vi "main OP600_V2.vi"() -> ()   [LabVIEW 2020]
uses:
  SubVI/OP600ZP_state.ctl
  <userlib>/PCAN Basic/Controls/BaudrateEenum.ctl
  <userlib>/PCAN Basic/Controls/Channel.ctl
  <userlib>/Alex.vi/FGV.ctl
  <vilib>/QMT/GDataBase for MySQL(tm)/MySQL/public/controls/DateType.ctl
  daa43a20-d466-48a4-bfb3-52e05527ce28.vi
  654b273e-591c-4045-8098-318fb337c7b6.vi
  e0de2198-bc36-4bc8-b1fb-14dde5ea0bb3.vi
  a5648d77-eeaa-4b2b-abe7-0ffab4b6f7d7.vi
  f79284c3-d1eb-48d9-b152-1e69b32bb97c.vi
  9714de12-b8a4-46e9-98c0-2b399b9db653.vi
  22d400d8-53c2-4810-82ae-66a3a2ac2ba8.vi
  51409799-00e2-4034-9917-3b3013219290.vi
  4ce1676d-84e0-48fa-8ffd-701686323251.vi
  OP500/VG/VG_progressBar.vi
  OP500/VG/VG_branche.vi
  SubVI/CheminDeBase.vi
  <vilib>/Utility/error.llb/Error Cluster From Error Code.vi
  VG/PN.vi
  VG/PackType.vi
  VG/IS30%.vi
  SubVI/OP600ZP_VGConf.vi
  VG/Ubatt.vi
  VG/OCV.vi
  VG/VG_ALIM.vi
  <vilib>/QMT/GDataBase for MySQL(tm)/MySQL/MySQLConnector.lvclass
  VG/VG_BT3564.vi
  <userlib>/Alex_Peak_lib/PEAK_lib_ALEX.lvlib
  <userlib>/PCAN Basic/PCANBasic.lvlib
panel:
  out "Revision":u32
  out "DeltaV30s":u32
  in  "cluster de sortie 2":T1
  in  "errin":errorcluster
  out "error out":errorcluster
  in  "errin":errorcluster
  in  "O/P/D":i8(slide)=1 scale=0.0..2.0
  out "OFF":bool
  out "PARK":bool=TRUE
  out "DRIVE":bool
  out "ST5520":refnum<visa-resource-name>
  out "BT3564":refnum<visa-resource-name>
  out "ALIM":refnum<visa-resource-name>
  in  "arrêt":bool
  out "BDD":T2
  out "VISA OUT":T3
  out "progression":dbl(slide) scale=0.0..30.0
  out "PN":string
  out "errout 2":errorcluster={"status"=TRUE, "code"=0, "source"="PCAN_CHANNEL ILLEGAL"} caption="errout"
  out "errout":errorcluster caption="sortie d'erreur"
  out "STOP":bool
  out "TOP":string
  out "DRAW":picture
  # "COMMANDE"
  # "DRIVE"
  # "PARK"
  # "OFF"
  # "SCAN ____________________________"
  # "SEALING ____________________________"
  # "CONTI ____________________________"
  # "CAN BAT / VEH ____________________________"
  # "PARK ____________________________"
  # "ISO ____________________________"
  # "OCV ____________________________"
  # "CAPA ____________________________"
  # "PRECHARGE ____________________________"
  # "DCIR ____________________________"
  # "PARK 2  ____________________________"
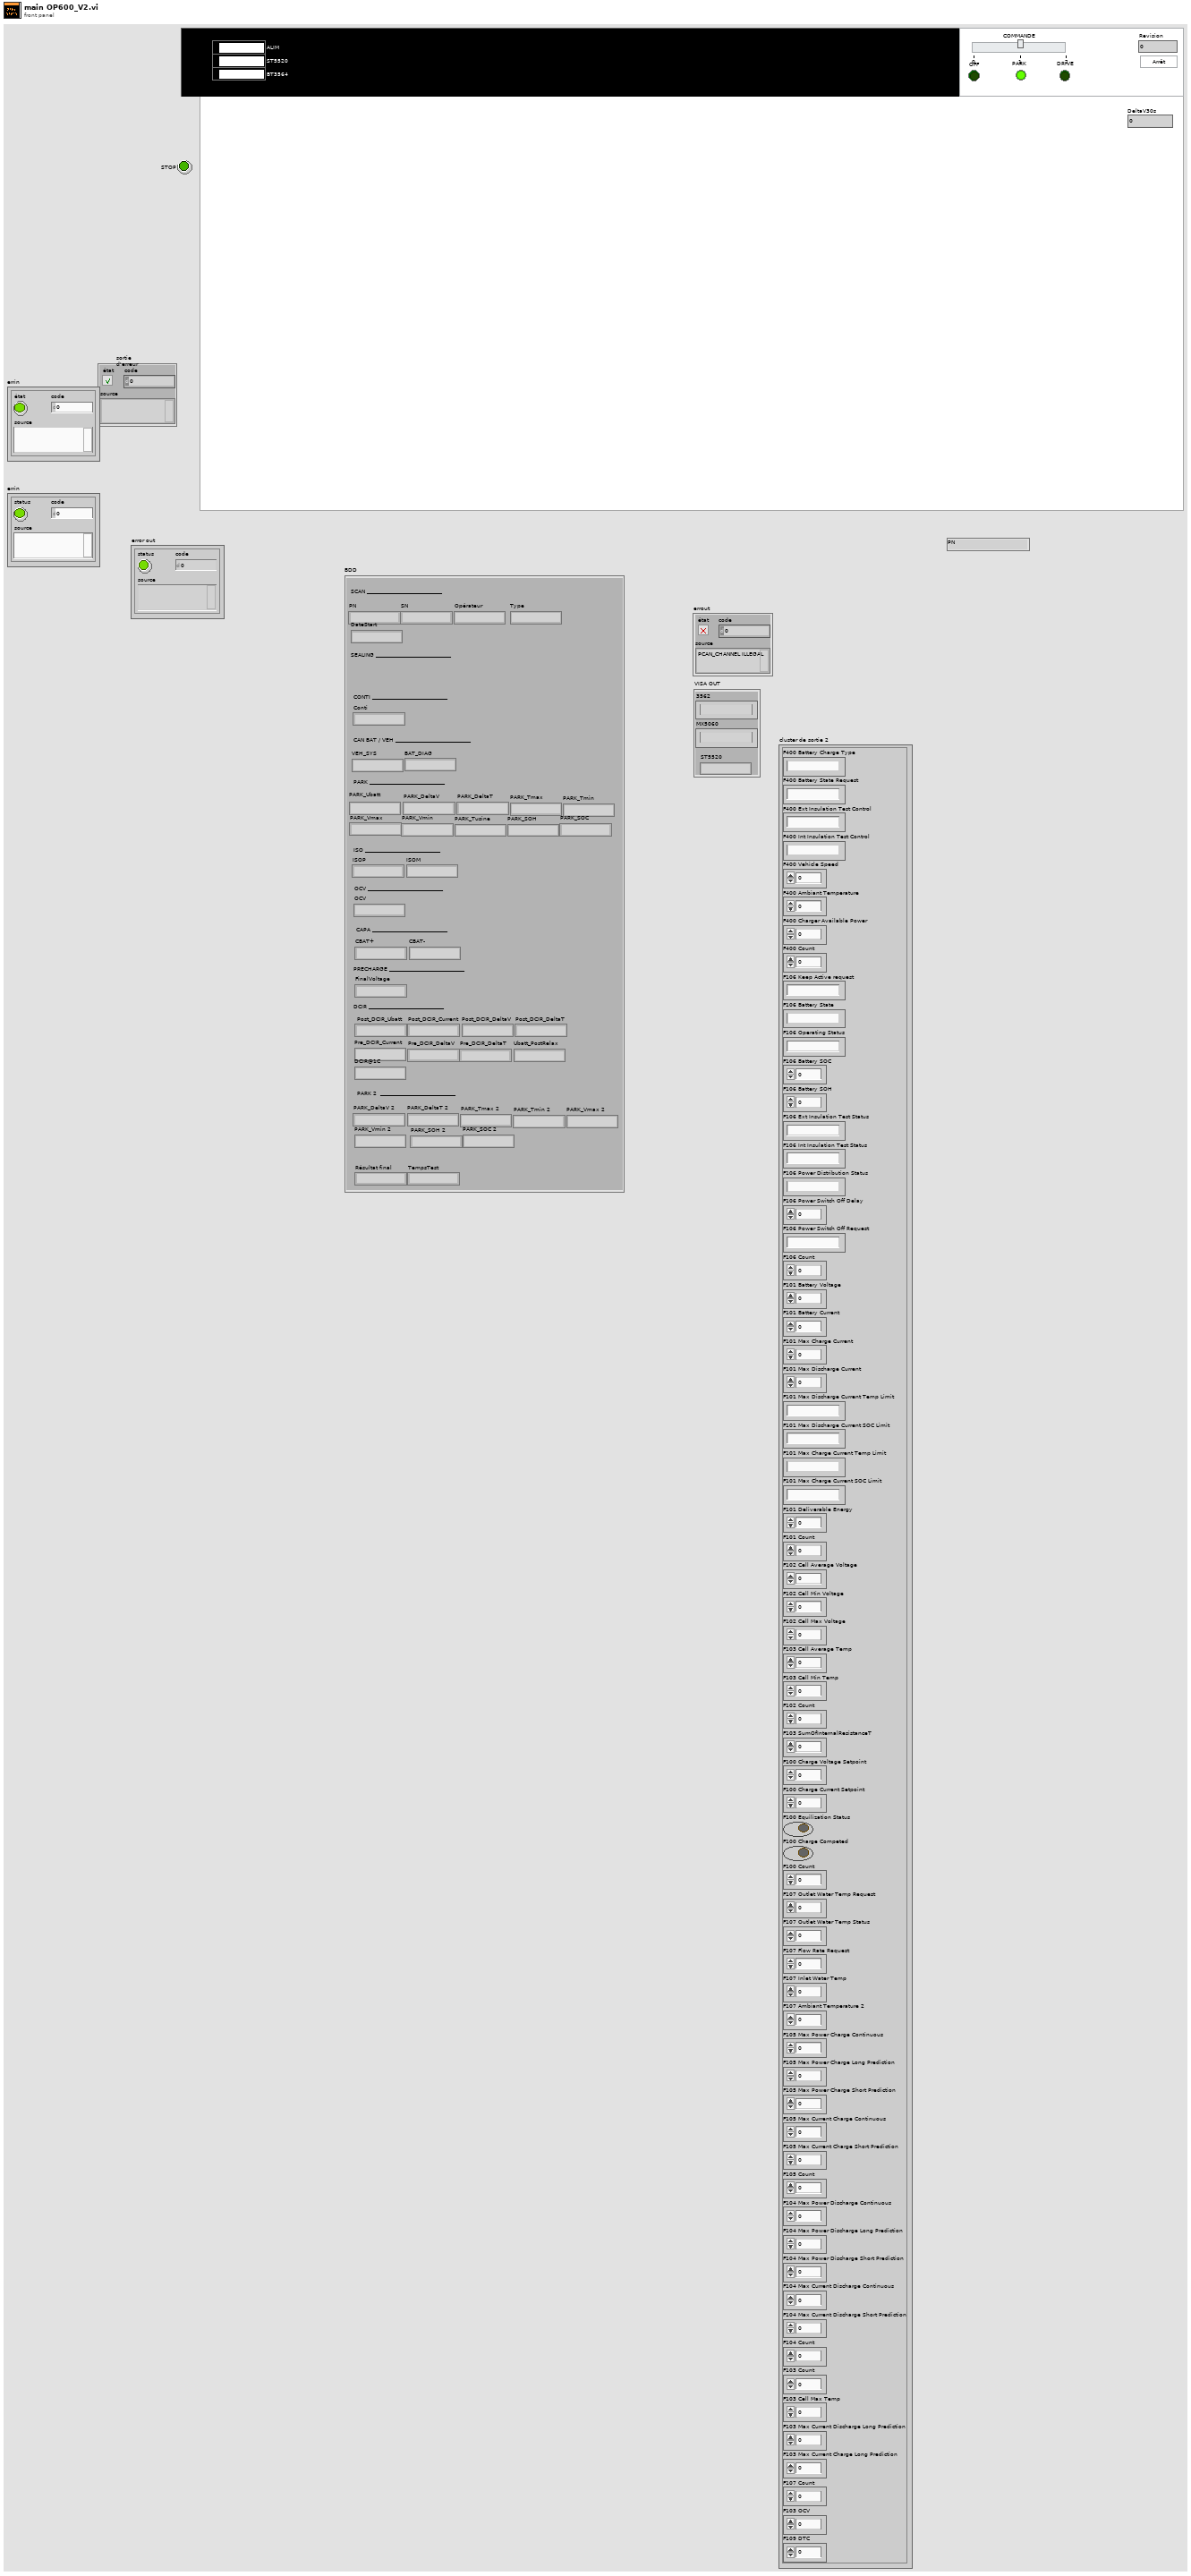
[diagram p1: front panel]
types:
  T1 = cluster{"F400 Battery Charge Type":string, "F400 Battery State Request":string, "F400 Ext Insulation Test Control":string, "F400 Int Insulation Test Control":string, "F400 Vehicle Speed":i32, "F400 Ambiant Temperature":i32, "F400 Charger Available Power":i32, "F400 Count":i32, "F106 Keep Active request":string, "F106 Battery State":string, "F106 Operating Status":string, "F106 Battery SOC":dbl, "F106 Battery SOH":dbl, "F106 Ext Insulation Test Status":string, "F106 Int Insulation Test Status":string, "F106 Power Distribution Status":string, "F106 Power Switch Off Delay":i32, "F106 Power Switch Off Request":string, "F106 Count":i32, "F101 Battery Voltage":u32, "F101 Battery Current":dbl, "F101 Max Charge Current":u32, "F101 Max Discharge Current":u32, "F101 Max Discharge Current Temp Limit":string, "F101 Max Discharge Current SOC Limit":string, "F101 Max Charge Current Temp Limit":string, "F101 Max Charge Current SOC Limit":string, "F101 Deliverable Energy":dbl, "F101 Count":u32, "F102 Cell Average Voltage":u32, "F102 Cell Min Voltage":u32, "F102 Cell Max Voltage":u32, "F103 Cell Average Temp":i32, "F103 Cell Min Temp":i32, "F102 Count":u32, "F103 SumOfInternalResistanceT":i32, "F100 Charge Voltage Setpoint":i32, "F100 Charge Current Setpoint":dbl, "F100 Equilization Status":bool, "F100 Charge Competed":bool, "F100 Count":i32, "F107 Outlet Water Temp Request":i32, "F107 Outlet Water Temp Status":i32, "F107 Flow Rate Request":i32, "F107 Inlet Water Temp":i32, "F107 Ambiant Temperature 2":i32, "F105 Max Power Charge Continuous":i32, "F105 Max Power Charge Long Prediction":i32, "F105 Max Power Charge Short Prediction":i32, "F105 Max Current Charge Continuous":i32, "F105 Max Current Charge Short Prediction":i32, "F105 Count ":i32, "F104 Max Power Discharge Continuous":i32, "F104 Max Power Discharge Long Prediction":i32, "F104 Max Power Discharge Short Prediction":i32, "F104 Max Current Discharge Continuous":i32, "F104 Max Current Discharge Short Prediction":i32, "F104 Count ":i32, "F103 Count":i32, "F103 Cell Max Temp":i32, "F103 Max Current Discharge Long Prediction":i32, "F103 Max Current Charge Long Prediction":i32, "F107 Count":i32, "F103 OCV":i32, "F109 DTC":i32}
  T2 = cluster{"PN":string, "SN":string, "Opérateur":string, "Type":string, "DateStart":string, "Conti":string, "VEH_SYS":string, "BAT_DIAG":string, "PARK_Ubatt":string, "PARK_DeltaV":string, "PARK_DeltaT":string, "PARK_Tmax":string, "PARK_Tmin":string, "PARK_Vmax":string, "PARK_Vmin":string, "PARK_Tusine":string, "PARK_SOH":string, "PARK_SOC":string, "ISOP":string, "ISOM":string, "OCV":string, "CBAT+":string, "CBAT-":string, "FinalVoltage":string, "Post_DCIR_Ubatt":string, "Post_DCIR_Current":string, "Post_DCIR_DeltaV":string, "Post_DCIR_DeltaT ":string, "Pre_DCIR_Current":string, "Pre_DCIR_DeltaV":string, "Pre_DCIR_DeltaT":string, "Ubatt_PostRelax":string, "DCIR@1C":string, "PARK_DeltaV 2":string, "PARK_DeltaT 2":string, "PARK_Tmax 2":string, "PARK_Tmin 2":string, "PARK_Vmax 2":string, "PARK_Vmin 2":string, "PARK_SOH 2":string, "PARK_SOC 2":string, "Résultat final":string, "TempsTest":string}
  T3 = cluster{"3562":string, "MX5060":string, "ST5520":string}
  T4 = typedef "PCANBasic.lvlib/Channel.ctl" = enum16{"PCAN_NONEBUS", "not used1", "not used2", "not used3", "not used4", "not used5", "not used6", "not used7", "not used8", "not used9", "not used10", "not used11", "not used12", "not used13", "not used14", "not used15", "not used16", "not used17", "not used18", "not used19", "not used20", "not used21", "not used22", "not used23", "not used24", "not used25", "not used26", "not used27", "not used28", "not used29", "not used30", "not used31", "not used32", "PCAN_ISABUS1", "PCAN_ISABUS2", "PCAN_ISABUS3", "PCAN_ISABUS4", "PCAN_ISABUS5", "PCAN_ISABUS6", "PCAN_ISABUS7", "PCAN_ISABUS8", "not used41", "not used42", "not used43", "not used44", "not used45", "not used46", "not used47", "not used48", "PCAN_DNGBUS1", "not used50", "not used51", "not used52", "not used53", "not used54", "not used55", "not used56", "not used57", "not used58", "not used59", "not used60", "not used61", "not used62", "not used63", "not used64", "PCAN_PCIBUS1", "PCAN_PCIBUS2", "PCAN_PCIBUS3", "PCAN_PCIBUS4", "PCAN_PCIBUS5", "PCAN_PCIBUS6", "PCAN_PCIBUS7", "PCAN_PCIBUS8", "not used73", "not used74", "not used75", "not used76", "not used77", "not used78", "not used79", "not used80", "PCAN_USBBUS1", "PCAN_USBBUS2", "PCAN_USBBUS3", "PCAN_USBBUS4", "PCAN_USBBUS5", "PCAN_USBBUS6", "PCAN_USBBUS7", "PCAN_USBBUS8", "Not used89", "Not used90", "Not used91", "Not used92", "Not used93", "Not used94", "Not used95", "Not used96", "PCAN_PCCBUS1", "PCAN_PCCBUS2"}
  T5 = typedef "PCANBasic.lvlib/BaudrateEenum.ctl" = enum16{"CAN_Baud_1M", "CAN_Baud_800K", "CAN_BAUD_500K", "CAN_BAUD_250K", "CAN_BAUD_125K", "CAN_BAUD_100K", "CAN_BAUD_95K", "CAN_BAUD_83K", "CAN_BAUD_50K", "CAN_BAUD_47K", "CAN_BAUD_33K", "CAN_BAUD_20K", "CAN_BAUD_10K", "CAN_BAUD_5K", "User Baudrate"}
  T6 = cluster{"PN":string, "Sealing":string, "Opérateur":string, "Conti":string, "OCV":string, "ISOP":string, "ISOM":string, "1_TCellmin":string, "1_TCellmax":string, "1_VCellmin":string, "1_VCellmax":string, "1_Nbmodule":string, "2_TCellmin":string, "2_TCellmax":string, "2_VCellmin":string, "2_VCellmax":string, "2_Nbmodule":string, "Résultat final":string, "Résultat final 2":string, "2_Nbmodule 2":string, "2_VCellmax 2":string, "2_VCellmin 2":string, "2_TCellmax 2":string, "Résultat final 3":string, "2_Nbmodule 3":string, "2_VCellmax 3":string, "2_VCellmin 3":string, "2_TCellmax 3":string, "2_TCellmin 2":string, "1_Nbmodule 2":string, "Résultat final 4":string, "2_Nbmodule 4":string, "2_VCellmax 4":string, "2_VCellmin 4":string, "2_TCellmax 4":string, "Résultat final 5":string, "2_Nbmodule 5":string, "2_VCellmax 5":string, "Résultat final 6":string, "2_Nbmodule 6":string, "2_VCellmax 6":string, "2_VCellmin 5":string, "2_TCellmax 5":string}
  T7 = typedef "OP600ZP_state.ctl" = enum16{"Null", "Demarrage", "Init", "Scan", "Sealing", "VAT", "Conti", "CAN Resistance", "Softs", "MCU", "Iso", "OCV", "DTC", "PreCharge", "DTC2", "PARK", "FIN_TEST", "PackVoltage", "Capacitance", "INTERLOOP", "Current + DCIR", "DataDyn", "Crash", "Next", "Comext"}
  T8 = typedef "FGV.ctl" = enum16{"GET", "SET", "RAZ"}
  T9 = typedef "imagedata.ctl" = cluster{"image type":i32, "image depth":i32, "image":u8[], "mask":u8[], "colors":u32[], "Rectangle":cluster{"left":i16, "top":i16, "right":i16, "bottom":i16}}
  T10 = typedef "MySQLVIEW.lvlib/MySQLConnector.lvclass/DateType.ctl" = enum16{"DATETIME", "DATE", "TIMESTAMP", "TIME", "YEAR (2 digits)", "YEAR (4 digits)"}
  T11 = cluster{string, string, string, string, string, string, string, string}
  T12 = cluster{"3564":string, "ALIM":string, "ST5520":string}
  T13 = cluster{string, string, string, string, string, string, string, string, string, string}
  T14 = cluster{"F101 Battery Voltage":u32, "F101 Battery Current":dbl, u32, i32, "F101 Battery Current":dbl, u32, i32, "F101 Battery Voltage":u32}
  T15 = cluster{string, string, string, string, string, string, string, string, string}
  T16 = cluster{"ID":u32, "MSGTYPE":u8, "LEN":u8, "DATA[0]":u8, "DATA[1]":u8, "DATA[2]":u8, "DATA[3]":u8, "DATA[4]":u8, "DATA[5]":u8, "DATA[6]":u8, "DATA[7]":u8}
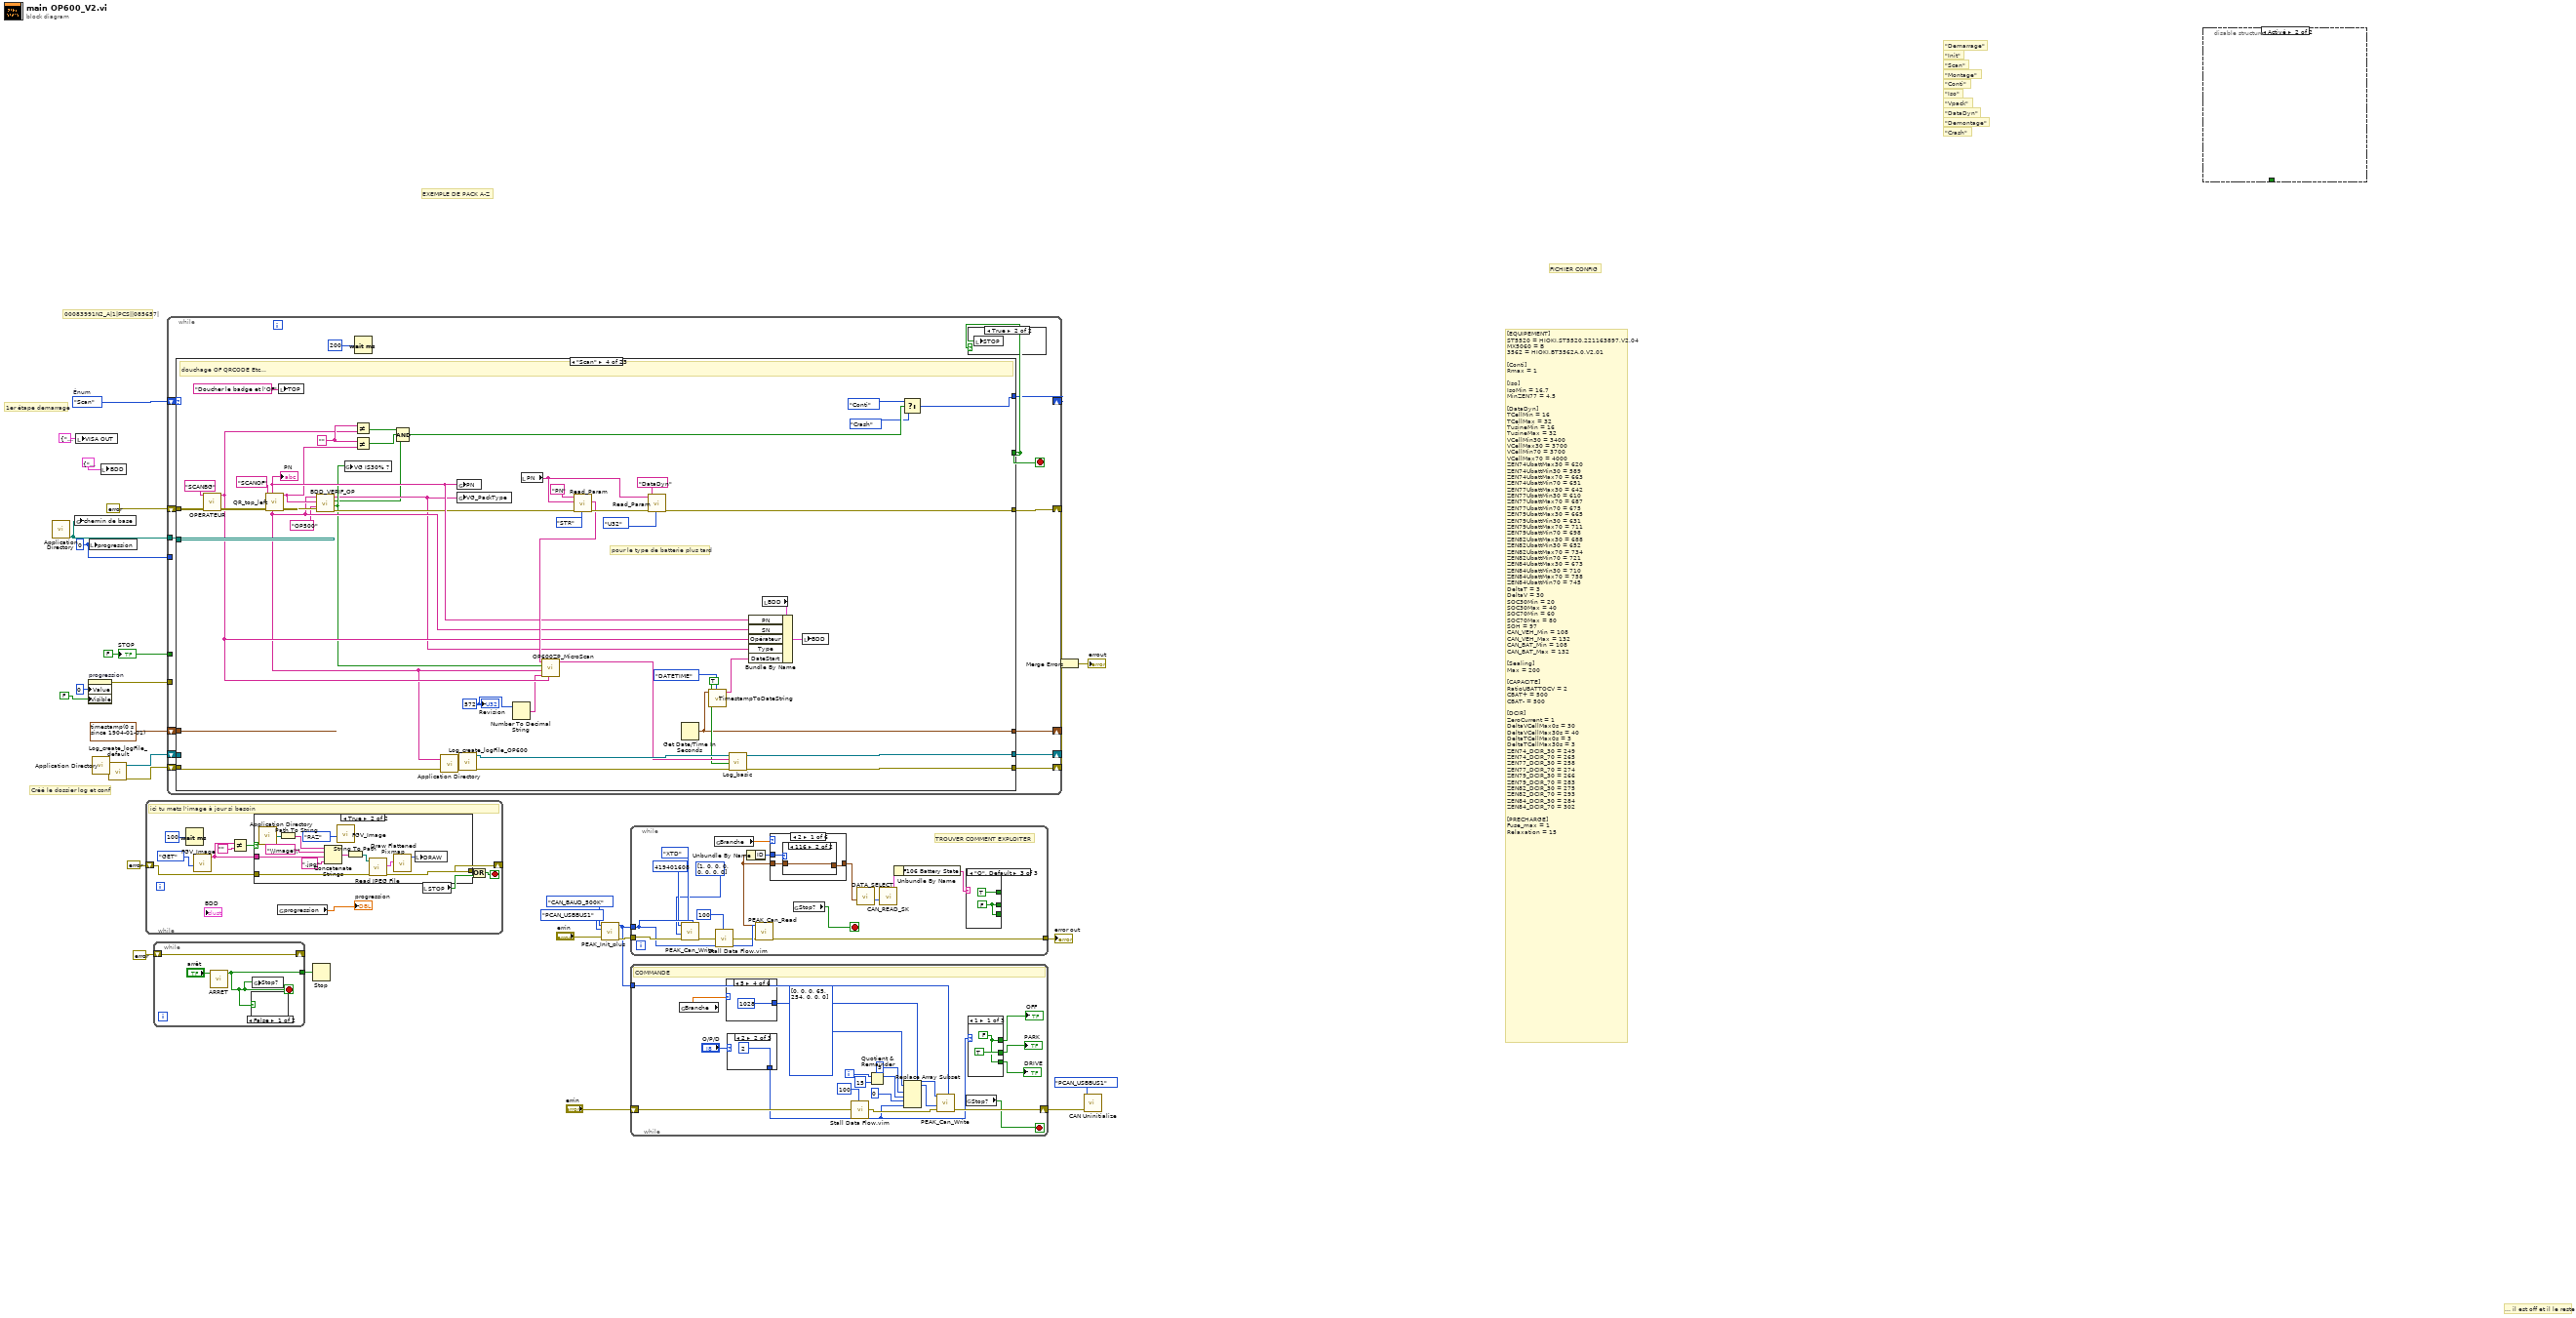
[diagram p0: block diagram]
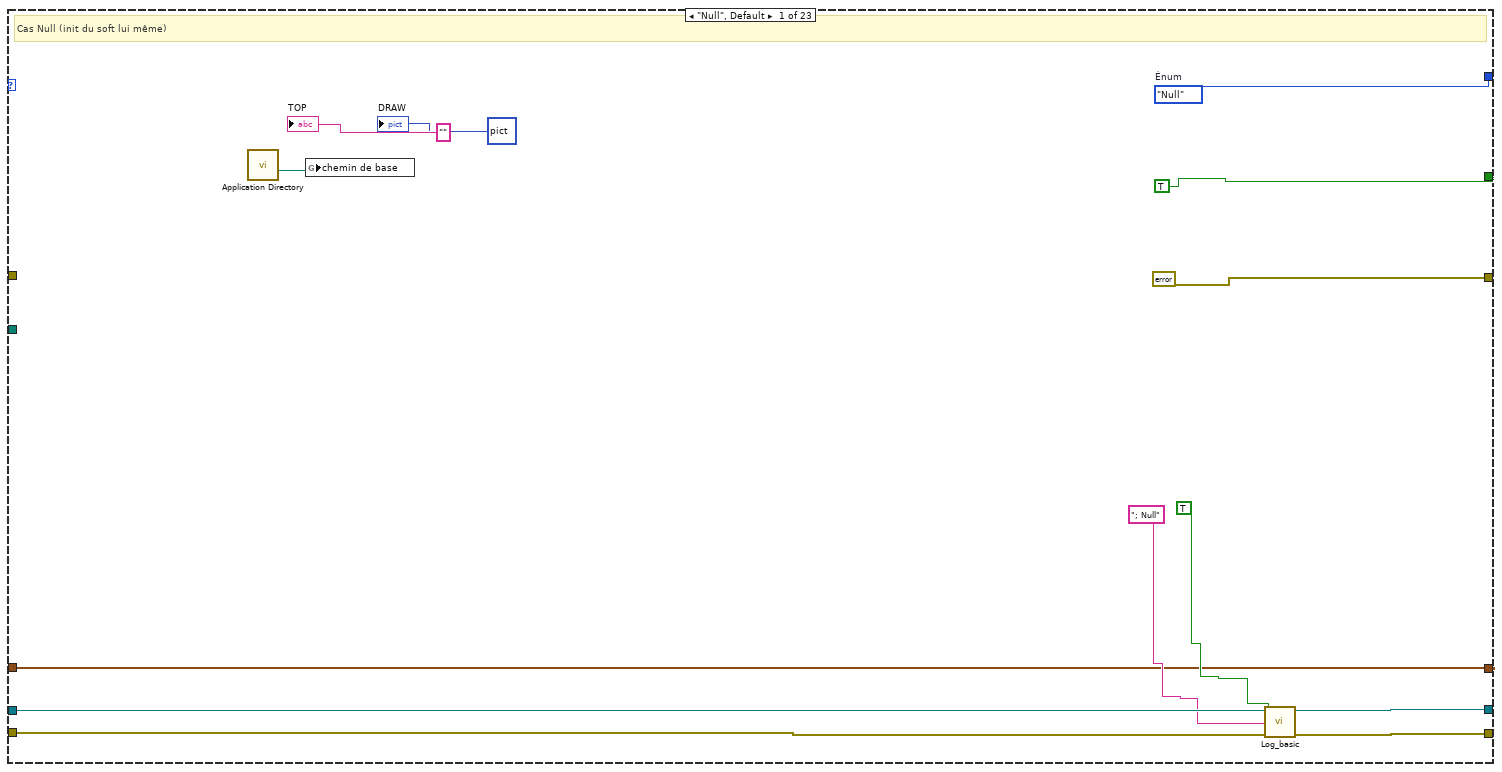
[diagram p2: hidden frame]
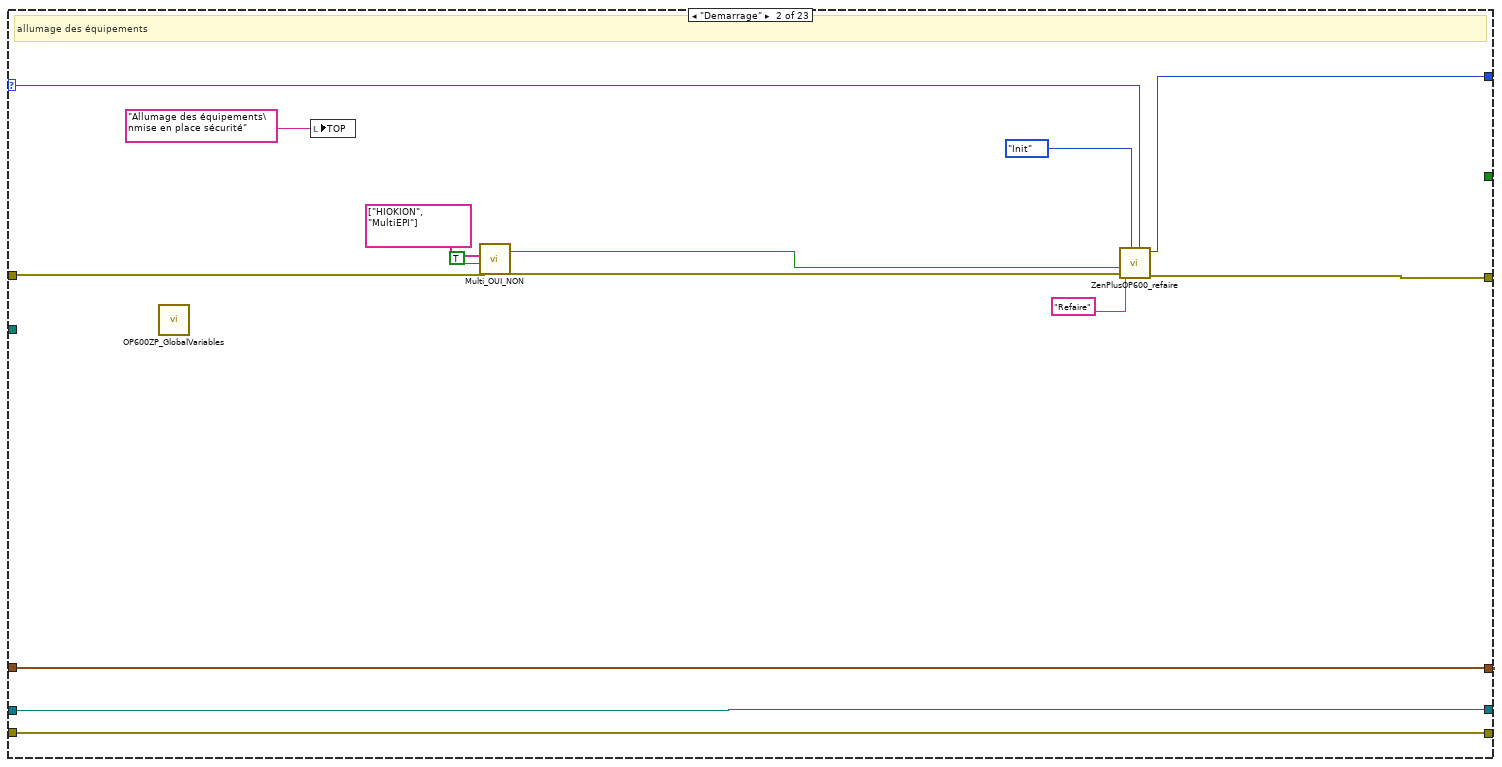
[diagram p3: hidden frame]
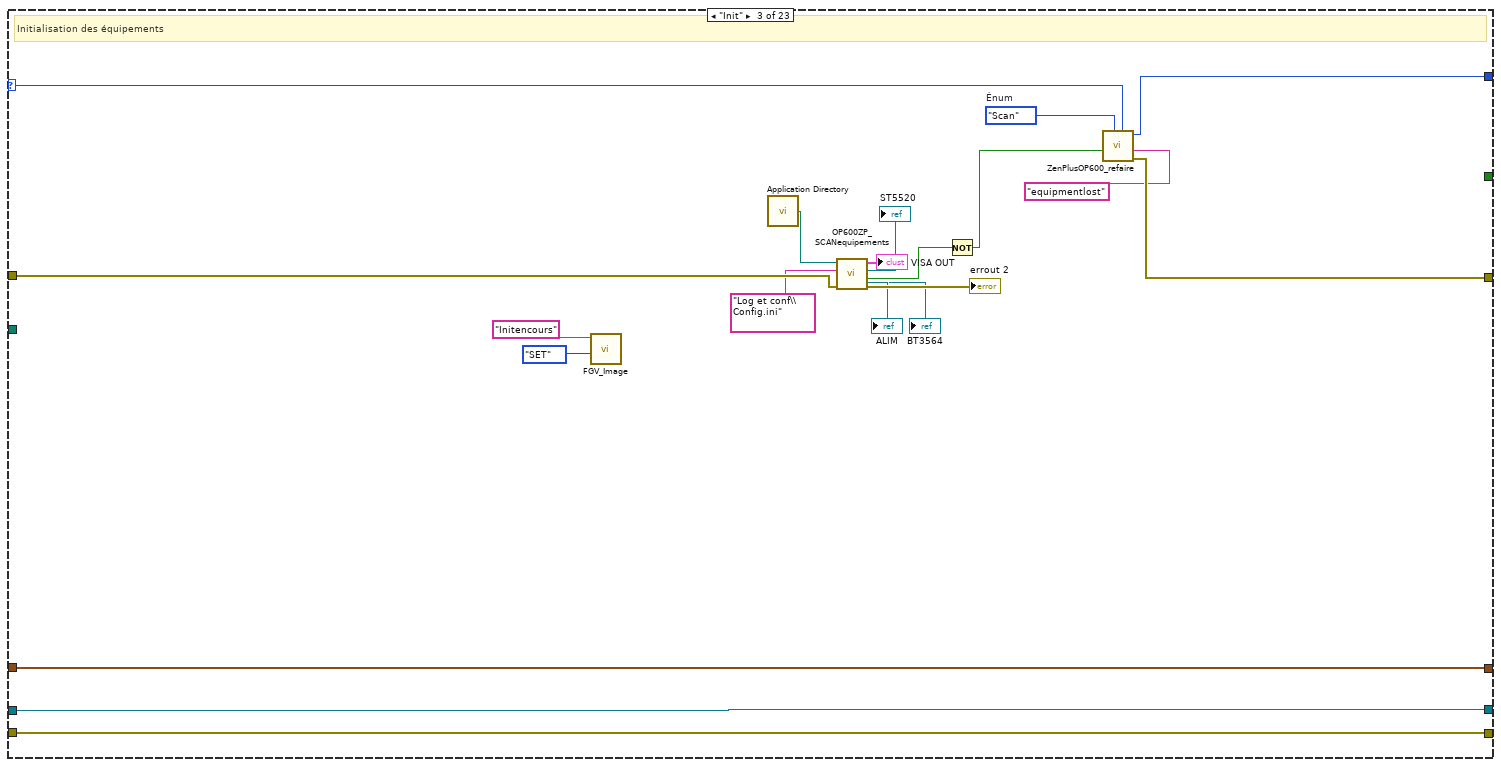
[diagram p4: hidden frame]
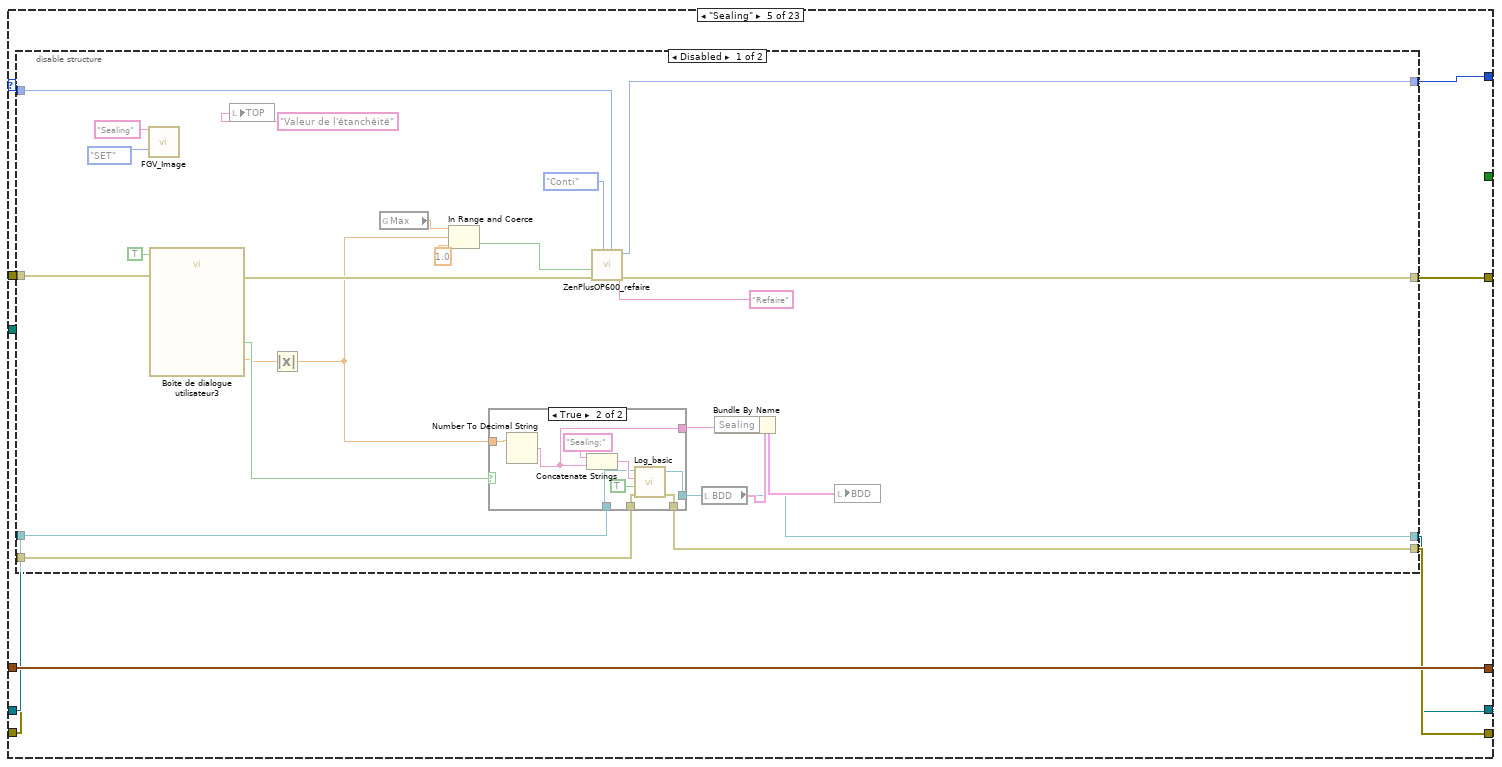
[diagram p5: hidden frame]
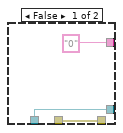
[diagram p6: hidden frame]
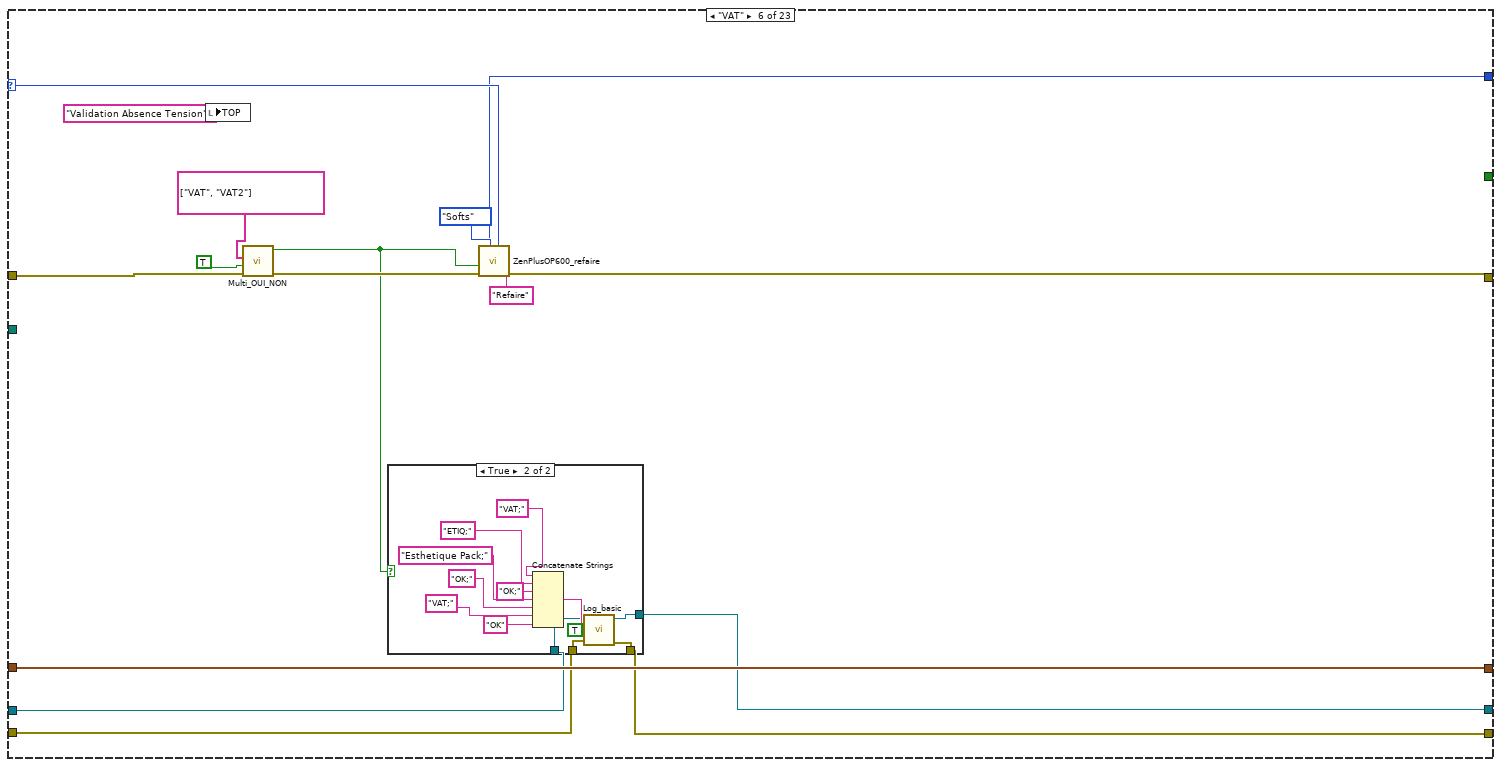
[diagram p8: hidden frame]
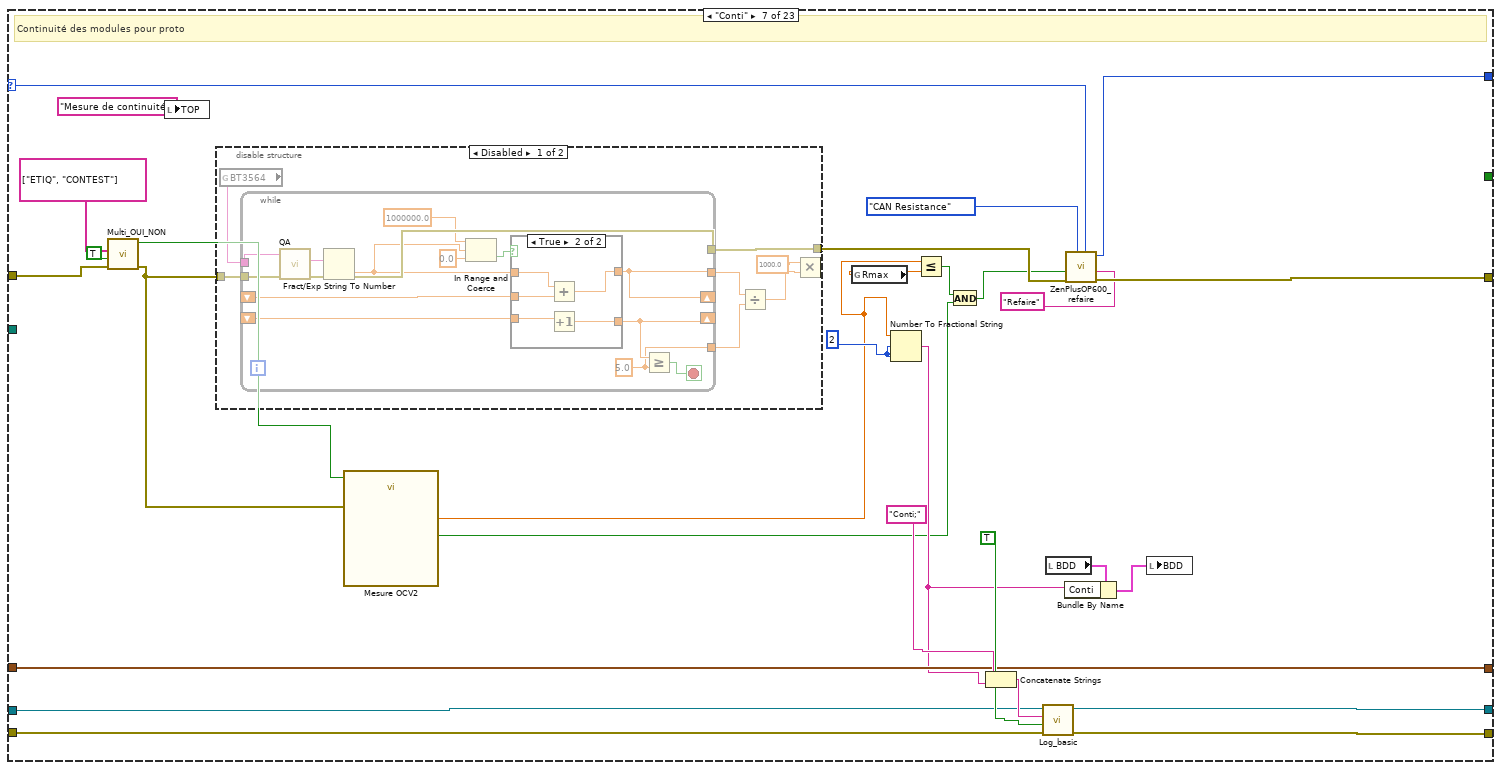
[diagram p10: hidden frame]
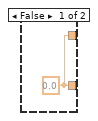
[diagram p11: hidden frame]
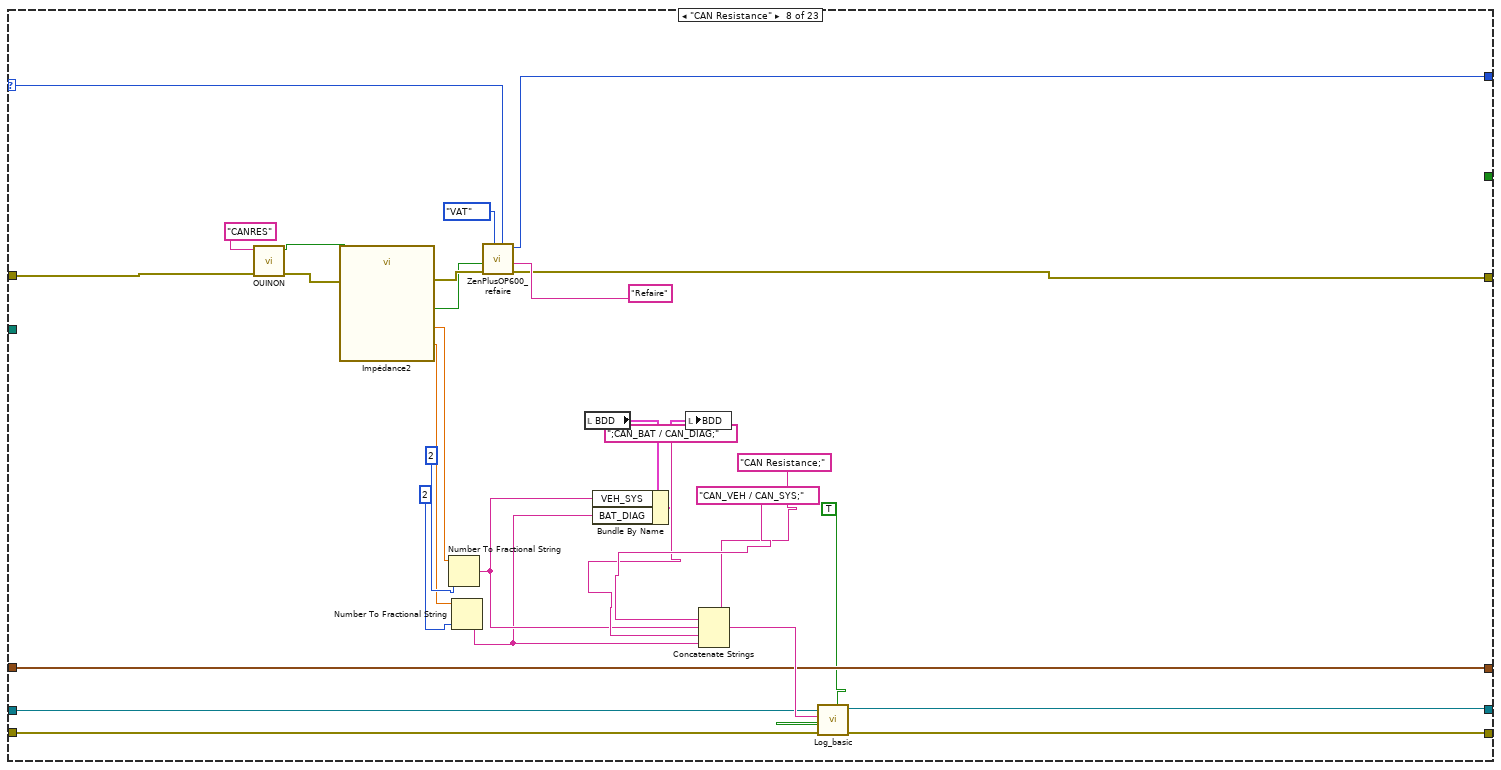
[diagram p13: hidden frame]
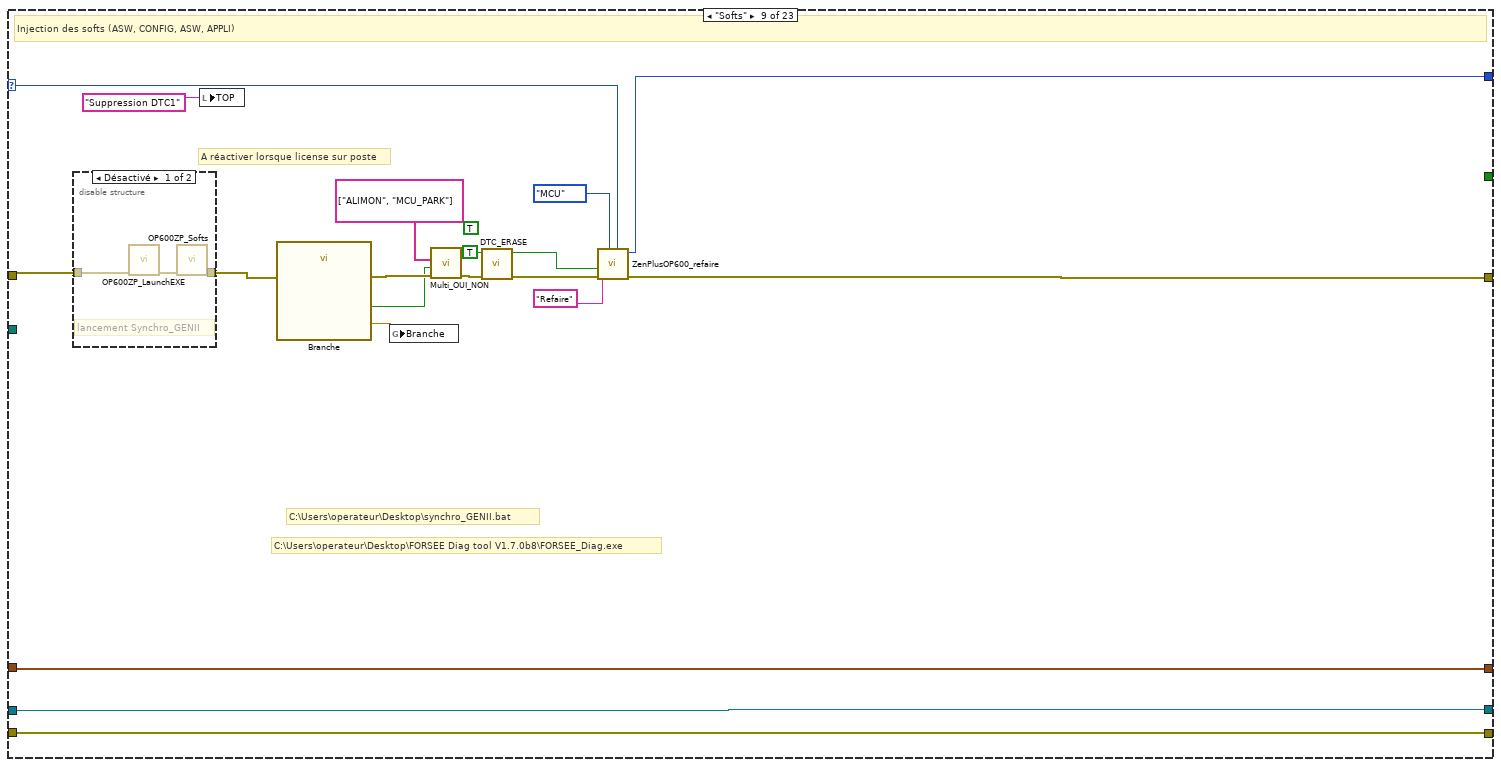
[diagram p14: hidden frame]
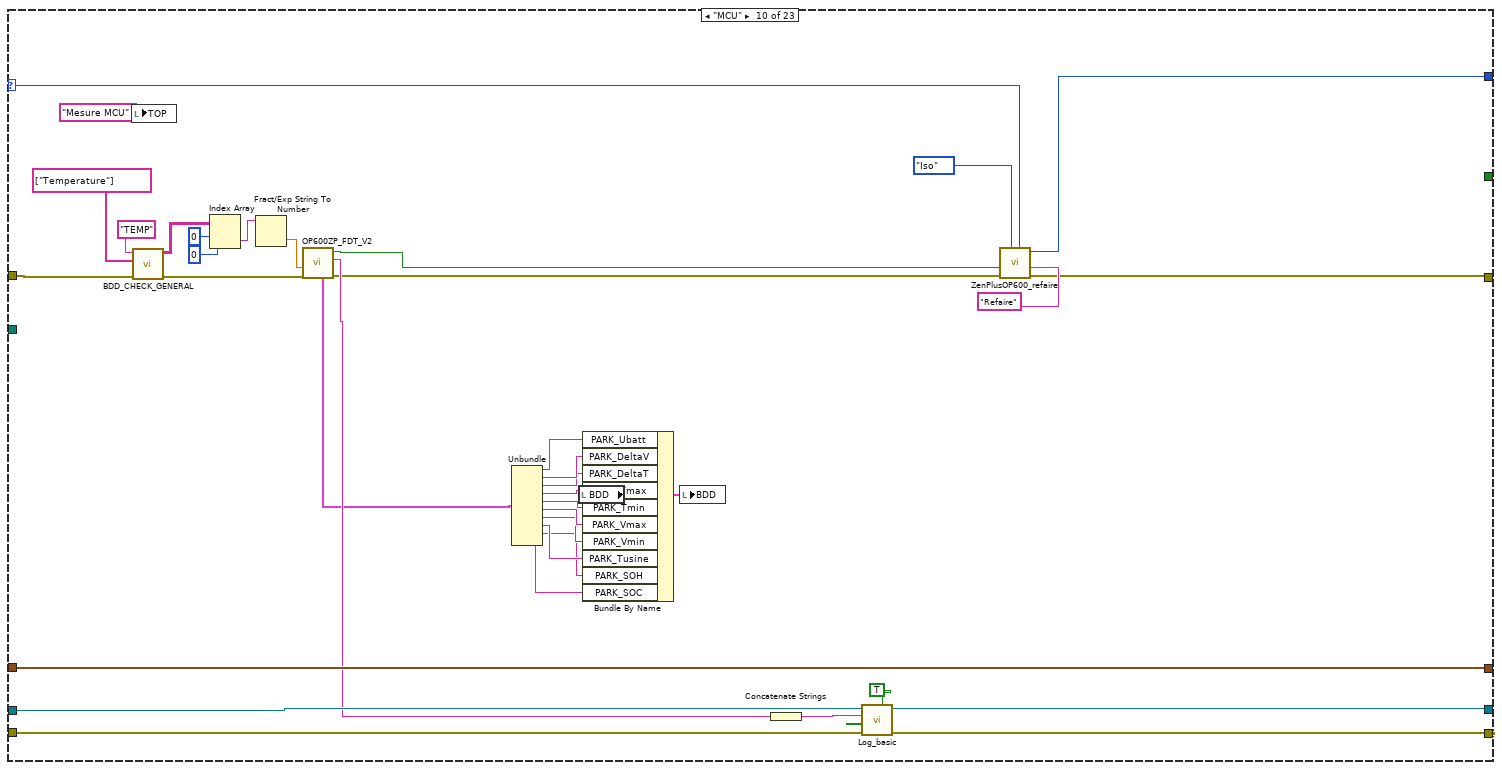
[diagram p16: hidden frame]
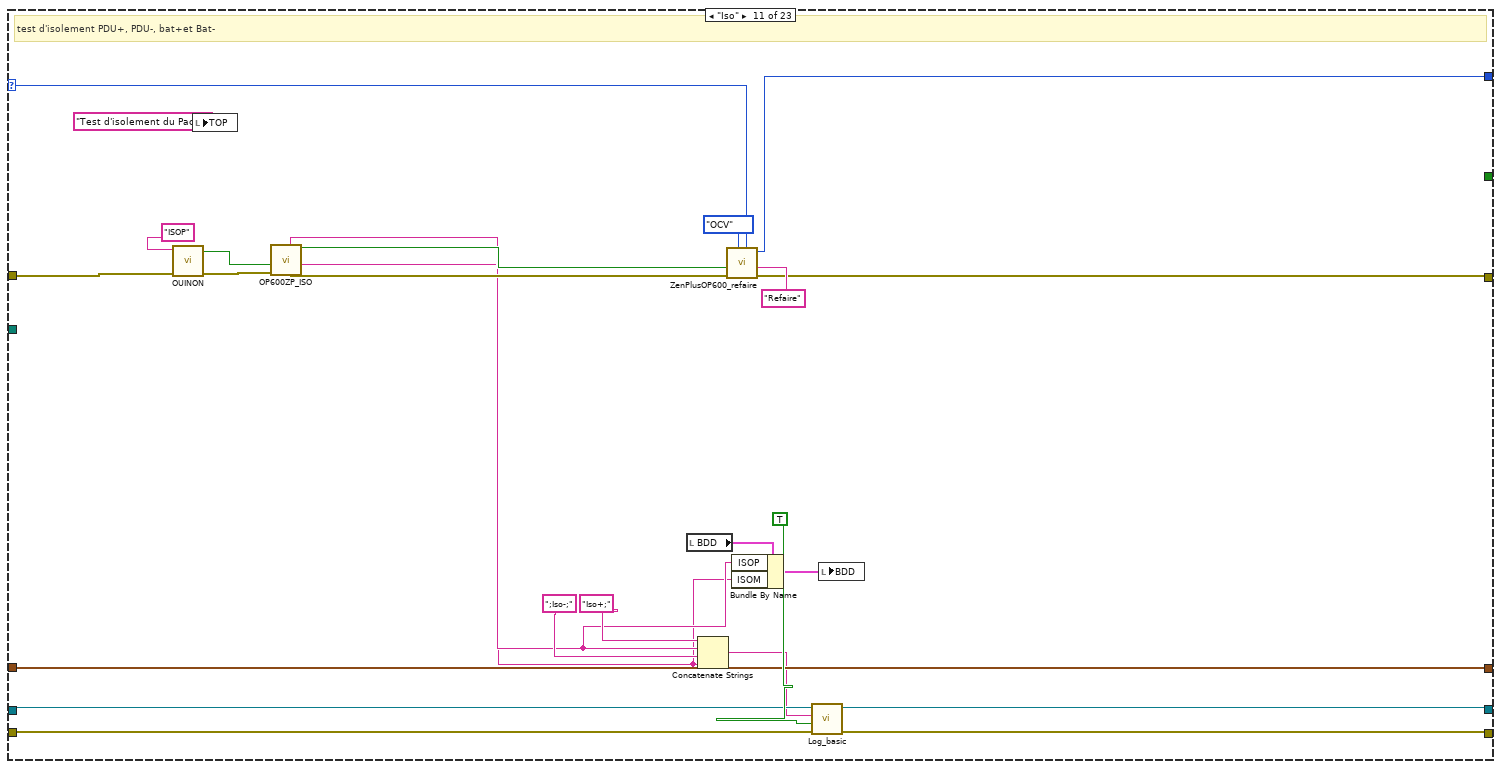
[diagram p17: hidden frame]
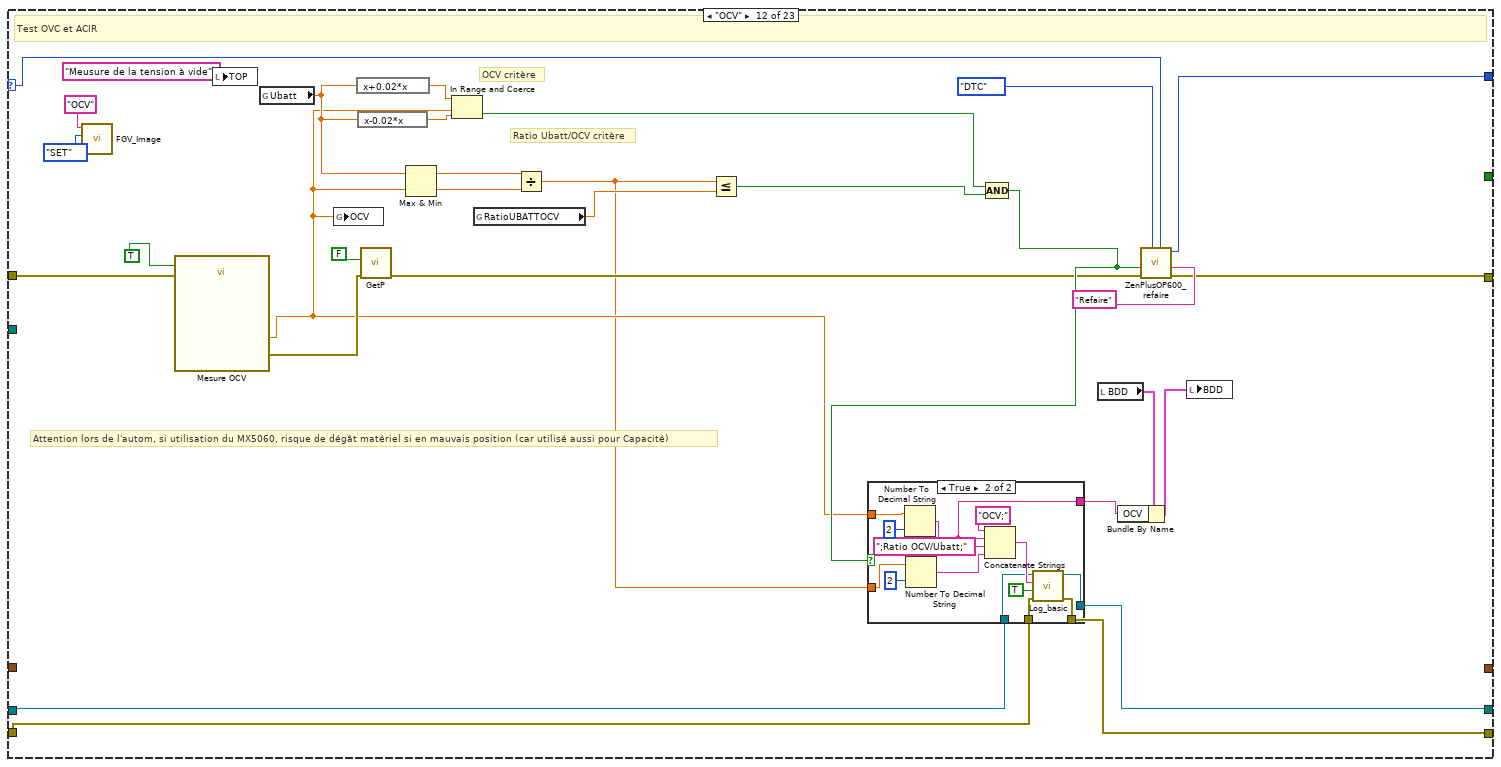
[diagram p18: hidden frame]
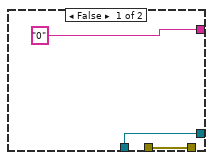
[diagram p19: hidden frame]
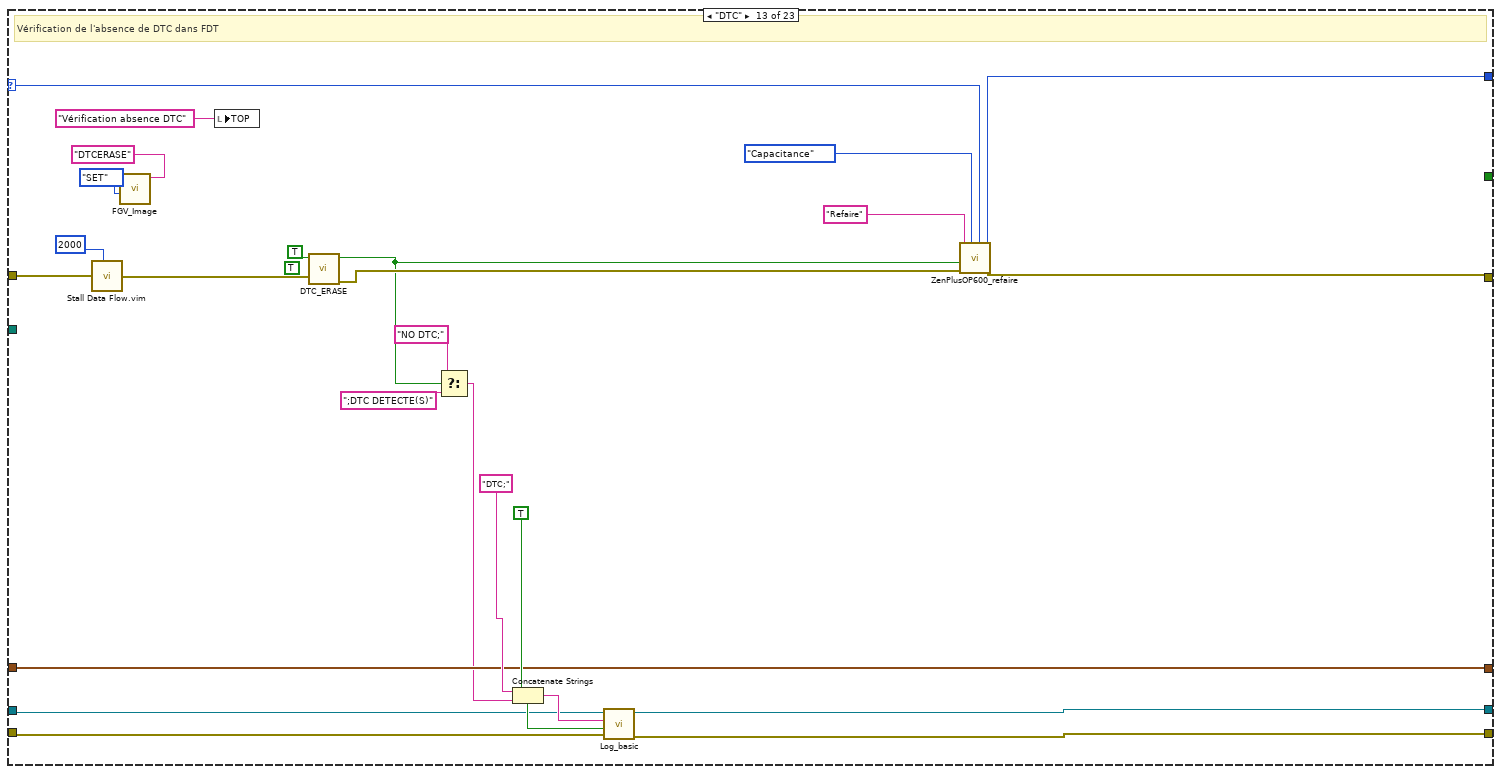
[diagram p20: hidden frame]
diagram:
  w19 = u8 0 ("progression")
  w13 = OP600ZP_state."Scan"  # Énum
  w25 = FALSE ("STOP")
  # "00083991N2_A|1|PCS||085657|"
  # "[EQUIPEMENT]\nST5520 = HIOKI,ST5520,221163897,V2.04\t\nMX5060 = B\n3562 = HIOKI,BT3562A,0,V2.01\n\n[Conti]\nRmax = 1\n\n[Iso]\nIsoMin = 16.7\nMinZEN77 = 4.5\n\n[DataDyn]\nTCellMin = 16\nTCellMax = 32\nTusineMin = 16\nTusineMax = 32\nVCellMin30 = 3400\nVCellMax30 = 3700\nVCellMin70 = 3700\nVCellMax70 = 4000\nZEN74UbattMax30 = 620\nZEN74UbattMin30 = 589\nZEN74UbattMax70 = 663\nZEN74UbattMin70 = 651\nZEN77UbattMax30 = 642\nZEN77UbattMin30 = 610\nZEN77UbattMax70 = 687\nZEN77UbattMin70 = 675\nZEN79UbattMax30 = 665\nZEN79UbattMin30 = 631\nZEN79UbattMax70 = 711\nZEN79UbattMin70 = 698\nZEN82UbattMax30 = 688\nZEN82UbattMin30 = 652\nZEN82UbattMax70 = 734\nZEN82UbattMin70 = 721\nZEN84UbattMax30 = 673\nZEN84UbattMin30 = 710\nZEN84UbattMax70 = 758\nZEN84UbattMin70 = 745\nDeltaT = 3\nDeltaV = 30\nSOC30Min = 20\nSOC30Max = 40\nSOC70Min = 60\nSOC70Max = 80\nSOH = 97\nCAN_VEH_Min = 108\nCAN_VEH_Max = 132\nCAN_BAT_Min = 108\nCAN_BAT_Max = 132\n\n[Sealing]\nMax = 200\n\n[CAPACITE]\nRatioUBATTOCV = 2\nCBAT+ = 500\nCBAT- = 500\n\n[DCIR]\nZeroCurrent = 1\nDeltaVCellMax0s = 30\nDeltaVCellMax30s = 40\nDeltaTCellMax0s = 3\nDeltaTCellMax30s = 3\nZEN74_DCIR_30 = 249\nZEN74_DCIR_70 = 265\nZEN77_DCIR_30 = 258\nZEN77_DCIR_70 = 274\nZEN79_DCIR_30 = 266\nZEN79_DCIR_70 = 283\nZEN82_DCIR_30 = 275\nZEN82_DCIR_70 = 293\nZEN84_DCIR_30 = 284\nZEN84_DCIR_70 = 302\n\n[PRECHARGE]\nFuse_max = 1\nRelaxation = 15"
  # "EXEMPLE DE PACK A-Z"
  # "FICHIER CONFIG"
  # "Créé le dossier log et conf"
  # "1er étape demarrage"
  # "\"Crash\""
  # "\"Demontage\""
  # "\"DataDyn\""
  # "\"Iso\""
  # "\"Montage\""
  # "\"Scan\""
  # "\"Init\""
  # "\"Demarrage\""
  # "\"Conti\""
  # "\"Vpack\""
  # "... il est off et il le reste"
  n1 = call <vilib>:"Application Directory.vi"() -> ("Application Directory"=w24:path)
  n2 = global write "CheminDeBase.vi" "chemin de base"(w24) -> ()
  n3 = local write "VISA OUT"(T3 {"3562"="", "MX5060"="", "ST5520"=""} ("VISA OUT")) -> ()
  n4 = property on="progression" class="Slide (strict)"("Value"=u8 0 ("progression"), "Visible"=FALSE) -> (error out=w17:errorcluster)  [unwired: 2 in, 1 out]
  n5 = local write "progression"(w19) -> ()
  n6 = call <vilib>:"Application Directory.vi"() -> ("Application Directory"=w22:path)
  n7 = local write "BDD"(T6 {"PN"="0", "Sealing"="0", "Opérateur"="0", "Conti"="0", "OCV"="0", "ISOP"="0", "ISOM"="0", "1_TCellmin"="0", "1_TCellmax"="0", "1_VCellmin"="0", "1_VCellmax"="0", "1_Nbmodule"="0", "2_TCellmin"="0", "2_TCellmax"="0", "2_VCellmin"="0", "2_VCellmax"="0", "2_Nbmodule"="0", "Résultat final"="0", "Résultat final 2"="0", "2_Nbmodule 2"="0", "2_VCellmax 2"="0", "2_VCellmin 2"="0", "2_TCellmax 2"="0", "Résultat final 3"="0", "2_Nbmodule 3"="0", "2_VCellmax 3"="0", "2_VCellmin 3"="0", "2_TCellmax 3"="0", "2_TCellmin 2"="0", "1_Nbmodule 2"="0", "Résultat final 4"="0", "2_Nbmodule 4"="0", "2_VCellmax 4"="0", "2_VCellmin 4"="0", "2_TCellmax 4"="0", "Résultat final 5"="0", "2_Nbmodule 5"="0", "2_VCellmax 5"="0", "Résultat final 6"="0", "2_Nbmodule 6"="0", "2_VCellmax 6"="0", "2_VCellmin 5"="0", "2_TCellmax 5"="0"} ("Cluster")) -> ()
  n8 = call <userlib>:"Log_create_logFile_default.vi"("appdir"=w22) -> ("errout"=w23:errorcluster, "Fichier à flux d'octets en sortie"=w26:refnum<file>)  [unwired: 9 in]
  n9 = while {
    shift-right: [w38] -> _
    shift-left: errorcluster {"status"=FALSE, "code"=0, "source"=""} ("error out") -> [w35]
    stop <- w36 stop-if-true
    # "ici tu mets l'image à jour si besoin"
    n10 = Wait (ms)(milliseconds to wait=u32 100 ("attente (ms)")) -> ()  [unwired: 1 out]
    n11 = call <userlib>:"FGV_Image.vi"("Énum"=FGV."GET") -> ("OUT"=w31:string)  [unwired: 10 in]
    n12 = Not Equal?(x=w31, y="") -> (x != y?=w32:bool)
    n13 = case shown="True" w32 {
      tunnel: [w40 w45] -> w38
      tunnel: w35 -> [w40 w44]
      tunnel: w31 -> [_ w43]
      frame False {
      }
      frame True {
        n14 = call <vilib>:"Application Directory.vi"() -> ("Application Directory"=w48:path)
        n15 = Path To String(path=w48) -> (string=w49:string)
        n16 = Concatenate Strings(w49, "\\Image\\" ("chaîne"), w43, ".jpg" ("chaîne")) -> (w47:string)
        n17 = call <userlib>:"FGV_Image.vi"("Énum"=FGV."RAZ") -> ()  [unwired: 10 in, 1 out]
        n18 = String To Path(string=w47) -> (path=w46:path)
        n19 = call <vilib>:"Read JPEG File.vi"("error in (no error)"=w44, "path to JPEG file"=w46) -> ("error out"=w45:errorcluster, "image data"=w52:T9)  [unwired: 7 in, 1 out]
        n20 = call <vilib>:"Draw Flattened Pixmap.vi"("image data"=w52) -> ("new picture"=w41:picture)  [unwired: 8 in]
        n21 = local write "DRAW"(w41) -> ()
      }
    }
    n22 = global read "VG_progressBar.vi" "progression"() -> (→"progression":dbl)
    n23 = local read "STOP"() -> (w37:bool)
    n24 = Or(x=w38, y=w37) -> (x .or. y?=w36:bool)
  }
  n25 = while {
    tunnel: [w53] -> w12
    shift-right: [w54] -> _
    shift-left: errorcluster {"status"=FALSE, "code"=0, "source"=""} ("error out") -> [w54]
    stop <- w53 stop-if-true
    n26 = call "ARRET.vi"("arrêt"="arrêt") -> ("T button?"=w53:bool)  [unwired: 10 in]
    n27 = case shown="False" w53 {
      frame False {
      }
      frame True {
        n28 = call <userlib>:"CAN Uninitialize.vi"() -> ()  [unwired: 9 in, 3 out]
      }
    }
    n29 = global write "VG_Stop" "Stop?"(w53) -> ()
  }
  n30 = while {
    shift-right: [w67] -> w28
    shift-left: errorcluster {"status"=FALSE, "code"=0, "source"=""} ("error out") -> [w58]
    shift-right: [w63] -> w27
    shift-left: w23 -> [w66]
    shift-right: [w64] -> _
    shift-left: w26 -> [w65]
    tunnel: w24 -> [w61]
    tunnel: w25 -> [_]
    shift-right: [w59] -> _
    shift-left: timestamp(0 s since 1904-01-01) ("seconds since 1Jan1904") -> [w60]
    tunnel: w19 -> [_]
    tunnel: w17 -> [_]
    shift-right: [w56] -> _
    shift-left: w13 -> [w57]
    stop <- w62 stop-if-true
    n31 = case shown="\"Scan\"" w57 {
      selector: w57 -> [_ w88 w109 _ w163 w213 w251 w301 w334 w371 w389 w412 w470 w505 w557 w643 w736 w793 w832 w855 _ _ w962]
      tunnel: w58 -> [_ w85 w112 w131 w169 w219 w242 w320 w331 w353 w390 w430 w462 w526 w551 w648 w756 w780 w824 w853 w881 w923 w959]
      tunnel: [errorcluster {"status"=FALSE, "code"=0, "source"=""} ("errin") w90 w111 w147 w161 w211 w256 w298 w335 w374 w394 w429 w479 w506 w555 w644 w737 w785 w816 w849 w880 w927 w961] -> w67
      tunnel: w66 -> [w77 w92 w115 w157 w166 w209 w263 w307 w338 w381 w405 w426 w475 w518 w562 w638 w740 w791 w830 w852 w908 w945 w965]
      tunnel: w65 -> [w78 w95 w114 _ w167 w207 w262 w305 w337 w380 w404 w428 w473 w516 w563 w636 w743 w792 w829 w850 w909 w946 w964]
      tunnel: [w75 w95 w114 w159 w164 w206 w261 w304 w337 w378 w403 w427 w472 w515 w560 w635 w742 w789 w826 w848 _ _ w956] -> w64
      tunnel: [w76 w92 w115 w160 w165 w208 w260 w306 w338 w379 w406 w425 w474 w517 w561 w637 w741 w788 w827 w851 w884 w926 w963] -> w63
      tunnel: [TRUE _ _ _ _ _ _ _ _ _ _ _ _ _ _ _ _ _ _ _ w910 _ _] -> w62
      tunnel: w61 -> [_ _ _ _ _ _ _ _ _ _ _ _ _ _ _ _ _ _ _ _ _ _ w960]
      tunnel: w60 -> [w72 w94 w113 _ w168 w215 w258 w303 w340 w377 w402 _ w471 w513 w559 w641 w757 w790 w828 _ _ _ w957]
      tunnel: [w72 w94 w113 w129 w168 w215 w258 w303 w340 w377 w402 _ w471 w513 w559 w641 w757 w790 w828 _ _ _ w958] -> w59
      tunnel: [w69 w87 w107 w132 w162 w212 w250 w299 w332 w369 w387 w410 w468 w503 w556 w640 w735 w787 w831 w854 OP600ZP_state."Crash" w925 w955] -> w56
      frame "Null", Default {
        w69 = OP600ZP_state."Null"  # Énum
        # "Cas Null (init du soft lui même)"
        n32 = call <vilib>:"Application Directory.vi"() -> ("Application Directory"=w81:path)
        n33 = global write "CheminDeBase.vi" "chemin de base"(w81) -> ()
        n34 = call <userlib>:"Log_basic.vi"("errin"=w77, "date?"=TRUE, "chaîne"="; Null", "in"=w78) -> ("sortie d'erreur"=w76:errorcluster, "refnum en sortie"=w75:refnum<file>)  [unwired: 6 in]
        "DRAW" <- picture data[5B] ("DRAW")
        "TOP" <- "" ("TOP")
      }
      frame "Demarrage" {
        # "allumage des équipements"
        n35 = call "OP600ZP_GlobalVariables.vi"() -> ()  [unwired: 12 in]
        n36 = local write "TOP"("Allumage des équipements\nmise en place sécurité" ("TOP")) -> ()
        n37 = call "Multi_OUI_NON.vi"("errin"=w85, "errinb"=TRUE, "Tableau"=string[] ["HIOKION", "MultiEPI"]) -> ("errout"=w84:errorcluster, "isok?"=w83:bool)  [unwired: 7 in]
        n38 = call "ZenPlusOP600_refaire.vi"("image"="Refaire", "Refaire"=w88, "Cas ok"=OP600ZP_state."Init" ("casOK"), "errin"=w84, "test ok ?"=w83) -> ("errout"=w90:errorcluster, "Next"=w87:T7)  [unwired: 5 in]
      }
      frame "Init" {
        w108 = OP600ZP_state."Scan"  # Énum
        # "Initialisation des équipements"
        n39 = call <userlib>:"FGV_Image.vi"("Énum"=FGV."SET", "IN"="Initencours") -> ()  [unwired: 9 in, 1 out]
        n40 = call <vilib>:"Application Directory.vi"() -> ("Application Directory"=w103:path)
        n41 = call "OP600ZP_SCANequipements.vi"("Errin"=w112, "Chaîne"="Log et conf\\Config.ini", "pathin"=w103) -> ("errout"=→"errout 2":errorcluster, "KO?"=w102:bool, "ST5520"=→"ST5520":refnum<visa-resource-name>, "VISA OUT"=→"VISA OUT":T12, "BT3564"=→"BT3564":refnum<visa-resource-name>, "ALIM"=→"ALIM":refnum<visa-resource-name>)  [unwired: 3 in]
        n42 = Not(x=w102) -> (.not. x?=w96:bool)
        n43 = call "ZenPlusOP600_refaire.vi"("image"="equipmentlost", "Refaire"=w109, "Cas ok"=w108, "test ok ?"=w96) -> ("errout"=w111:errorcluster, "Next"=w107:T7)  [unwired: 6 in]
      }
      frame "Scan" {
        w126 = u32 572 ("Revision")
        w152 = "" ("x")
        # "pour le type de batterie plus tard"
        # "douchage OF QRCODE Etc..."
        n44 = call <userlib>:"OPERATEUR.vi"("errin"=w131, "IN"="SCANBG") -> ("error out"=w151:errorcluster, "Dataout"=w134:string)  [unwired: 8 in]
        n45 = call <userlib>:"QR_top_left.vi"("errin"=w151, "image"="SCANOF") -> ("error out"=w125:errorcluster, "Réponse"=w123:string, "SN"=w122:string, "PN"=w133:string)  [unwired: 5 in, 1 out]
        "PN" <- w133
        n46 = local write "TOP"("Doucher le badge et l'OF" ("TOP")) -> ()
        n47 = call <userlib>:"BDD_VERIF_OP.vi"("errin"=w125, "N°OPVerif?"="OP500", "OF"=w123, "SN"=w122) -> ("error out"=w124:errorcluster, "IS30% ?"=w120:bool, "Continue?"=w116:bool, "TYPE"=w119:string)  [unwired: 4 in]
        n48 = global write "IS30%.vi" "VG IS30% ?"(w120) -> ()
        n49 = Not Equal?(x=w152, y=w134) -> (x != y?=w117:bool)
        n50 = Not Equal?(x=w152, y=w123) -> (x != y?=w118:bool)
        n51 = Compound Arithmetic op=AND ("Opérateur arithmétique")(w117, w118, w116) -> (w140:bool)
        n52 = call <vilib>:"Application Directory.vi"() -> ("Application Directory"=w158:path)
        n53 = global write "PN.vi" "PN"(w133) -> ()
        n54 = global write "PackType.vi" "VG_PackType"(w119) -> ()
        n55 = call "Log_create_logFile_OP600.vi"("errin"=w157, "toute l'expression"=w122, "Application Directory"=w158) -> ("sortie d'erreur"=w155:errorcluster, "Fichier à flux d'octets en sortie"=w156:refnum<file>)  [unwired: 7 in]
        n56 = Number To Decimal String(number=w126) -> (decimal integer string=w130:string)  [unwired: 1 in]
        n57 = local read "PN"() -> (w143:string)
        n58 = call <userlib>:"Read_Param.vi"("Énum"=enum16{"STR", "DBL", "U32"}."STR", "errin"=w124, "section"=w143, "key"="PN") -> ("error out"=w146:errorcluster, "str"=w142:string)  [unwired: 3 in, 3 out]
        n59 = call "OP600ZP_MicroScan.vi"("Dataout"=w134, "Rev"=w130, "SN"=w122, "Oui"=w120, "str"=w142) -> ("Chaîne"=w154:string)  [unwired: 6 in]
        n60 = call <userlib>:"Read_Param.vi"("Énum"=enum16{"STR", "DBL", "U32"}."U32", "errin"=w146, "section"="DataDyn", "key"=w143) -> ("error out"=w147:errorcluster)  [unwired: 3 in, 4 out]
        n61 = Get Date/Time In Seconds() -> (seconds since 1Jan1904=w129:timestamp)
        n62 = call <vilib>:"TimestampToDateString.vi"("dateType"=DateType."DATETIME", "timestamp in"=w129) -> ("dateString"=w128:string)  [unwired: 8 in, 1 out]
        n63 = call <userlib>:"Log_basic.vi"("errin"=w155, "date?"=TRUE, "chaîne"=w154, "in"=w156) -> ("sortie d'erreur"=w160:errorcluster, "refnum en sortie"=w159:refnum<file>)  [unwired: 6 in]
        n64 = local read "BDD"() -> (w136:T2)
        n65 = Bundle By Name(cluster=w136, "PN"=w133, "SN"=w122, "Opérateur"=w134, "Type"=w119, "DateStart"=w128) -> (w135:T2)
        n66 = local write "BDD"(w135) -> ()
        n67 = Select ("Sélectionner")(t=OP600ZP_state."Conti" ("Énum"), s=w140, f=OP600ZP_state."Crash" ("cas faux")) -> (s? t:f=w132:T7)
        "Revision" <- w126
      }
      frame "Sealing" {
        n68 = disable-structure shown="Disabled" {
          disable-tunnel: w169 -> [w193 _]
          disable-tunnel: w167 -> [w186 _]
          disable-tunnel: w166 -> [w185 _]
          disable-tunnel: [w184 _] -> w165
          disable-tunnel: [w183 _] -> w164
          disable-tunnel: w163 -> [w178 _]
          disable-tunnel: [w177 _] -> w162
          disable-tunnel: [w174 _] -> w161
          frame Disabled {
            n69 = call <userlib>:"FGV_Image.vi"("Énum"=FGV."SET", "IN"="Sealing") -> ()  [unwired: 9 in, 1 out]
            n70 = call "Boîte de dialogue utilisateur3"("Enable"=TRUE, "error in (no error)"=w193) -> ("Étenchéité"=w171:dbl, "OK"=w173:bool, "error out"=w175:errorcluster)  [unwired: 15 in]
            n71 = local write "TOP"("Valeur de l'étanchéité" ("TOP")) -> ()
            n72 = Absolute Value(x=w171) -> (abs(x)=w170:dbl)
            n73 = global read "OP600ZP_VGConf.vi" "Max"() -> (w176:dbl)
            n74 = In Range and Coerce(upper limit=w176, x=w170, lower limit=1.0 ("limite inférieure")) -> (In Range?=w190:bool)  [unwired: 1 out]
            n75 = case shown="True" w173 {
              tunnel: [w194 w202] -> w183
              tunnel: w170 -> [_ w201]
              tunnel: ["0" w200] -> w187
              tunnel: w186 -> [w194 w199]
              tunnel: w185 -> [w195 w198]
              tunnel: [w195 w197] -> w184
              frame False {
              }
              frame True {
                n76 = Number To Decimal String(number=w201) -> (decimal integer string=w200:string)  [unwired: 1 in]
                n77 = Concatenate Strings("Sealing;" ("chaîne"), w200) -> (w204:string)
                n78 = call <userlib>:"Log_basic.vi"("errin"=w198, "date?"=TRUE, "chaîne"=w204, "in"=w199) -> ("sortie d'erreur"=w197:errorcluster, "refnum en sortie"=w202:refnum<file>)  [unwired: 6 in]
              }
            }
            n79 = call "ZenPlusOP600_refaire.vi"("image"="Refaire", "Refaire"=w178, "Cas ok"=OP600ZP_state."Conti", "errin"=w175, "test ok ?"=w190) -> ("errout"=w174:errorcluster, "Next"=w177:T7)  [unwired: 5 in]
            n80 = local read "BDD"() -> (w189:T2)
            n81 = Bundle By Name(cluster=w189, "Sealing"=w187) -> (w188:T2)
            n82 = local write "BDD"(w188) -> ()
          }
          frame Enabled {
          }
        }
      }
      frame "VAT" {
        n83 = local write "TOP"("Validation Absence Tension" ("TOP")) -> ()
        n84 = call "Multi_OUI_NON.vi"("errin"=w219, "errinb"=TRUE, "Tableau"=string[] ["VAT", "VAT2"]) -> ("errout"=w216:errorcluster, "isok?"=w210:bool)  [unwired: 7 in]
        n85 = case shown="True" w210 {
          tunnel: [w223 w234] -> w208
          tunnel: w209 -> [w223 w233]
          tunnel: [w222 w232] -> w206
          tunnel: w207 -> [w222 w231]
          frame False {
          }
          frame True {
            n86 = Concatenate Strings("VAT;" ("chaîne"), "ETIQ;" ("chaîne"), "OK;" ("chaîne"), "Esthetique Pack;" ("chaîne"), "OK;" ("chaîne"), "VAT;" ("chaîne"), "OK" ("chaîne")) -> (w235:string)
            n87 = call <userlib>:"Log_basic.vi"("errin"=w233, "date?"=TRUE, "chaîne"=w235, "in"=w231) -> ("sortie d'erreur"=w234:errorcluster, "refnum en sortie"=w232:refnum<file>)  [unwired: 6 in]
          }
        }
        n88 = call "ZenPlusOP600_refaire.vi"("image"="Refaire", "Refaire"=w213, "Cas ok"=OP600ZP_state."Softs" ("casOK"), "errin"=w216, "test ok ?"=w210) -> ("errout"=w211:errorcluster, "Next"=w212:T7)  [unwired: 5 in]
      }
      frame "Conti" {
        w249 = i16 2 ("largeur (-)")
        # "Continuité des modules pour proto"
        n89 = call "Multi_OUI_NON.vi"("errin"=w242, "errinb"=TRUE, "Tableau"=string[] ["ETIQ", "CONTEST"]) -> ("errout"=w241:errorcluster, "isok?"=w238:bool)  [unwired: 7 in]
        n90 = local write "TOP"("Mesure de continuité" ("TOP")) -> ()
        n91 = disable-structure shown="Disabled" {
          disable-tunnel: [w268 _] -> w247
          disable-tunnel: w241 -> [w266 _]
          frame Disabled {
            n92 = global read "VG_BT3564.vi" "BT3564"() -> (w267:string)
            n93 = while {
              tunnel: w266 -> [w286]
              shift-right: [w282] -> _
              shift-left: _ -> [w284]
              tunnel: [w282] -> w272
              tunnel: w267 -> [w283]
              shift-right: [w279] -> _
              shift-left: _ -> [w281]
              tunnel: [w278] -> w271
              tunnel: [w277] -> w268
              stop <- w280 stop-if-true
              w278 = 5.0 ("y")
              n94 = call "QA.vi"("ERRIN"=w286, 10:w283) -> ("ERROUT"=w277:errorcluster, "DATAOUT"=w285:string)  [unwired: 8 in]
              n95 = Fract/Exp String To Number(string=w285) -> (number=w274:dbl)  [unwired: 3 in, 1 out]
              n96 = In Range and Coerce(upper limit=1000000.0 ("limite supérieure"), x=w274, lower limit=0.0 ("limite inférieure")) -> (In Range?=w276:bool)  [unwired: 1 out]
              n97 = case shown="True" w276 {
                tunnel: w284 -> [_ w292]
                tunnel: [w287 w291] -> w282
                tunnel: w274 -> [_ w290]
                tunnel: w281 -> [_ w289]
                tunnel: [w287 w288] -> w279
                frame False {
                  w287 = 0.0
                }
                frame True {
                  n98 = Add(x=w290, y=w292) -> (x+y=w291:dbl)
                  n99 = Increment(x=w289) -> (x+1=w288:dbl)
                }
              }
              n100 = Greater Or Equal?(x=w279, y=w278) -> (x >= y?=w280:bool)
            }
            n101 = Divide(x=w272, y=w271) -> (x/y=w270:dbl)
            n102 = Multiply(x=1000.0, y=w270) -> ()  [unwired: 1 out]
          }
          frame Enabled {
          }
        }
        n103 = call "Mesure OCV2"("Enable"=w238, "error in (no error)"=w241) -> ("Continuité relevée :"=w243:dbl, "OK"=w237:bool)  [unwired: 15 in, 1 out]
        n104 = global read "OP600ZP_VGConf.vi" "Rmax"() -> (w248:dbl)
        n105 = Number To Fractional String(number=w243, width (-)=w249, precision (6)=w249) -> (F-format string=w246:string)  [unwired: 1 in]
        n106 = Less Or Equal?(x=w243, y=w248) -> (x <= y?=w245:bool)
        n107 = And(x=w245, y=w237) -> (x .and. y?=w244:bool)
        n108 = Concatenate Strings("Conti;" ("chaîne"), w246) -> (w265:string)
        n109 = call <userlib>:"Log_basic.vi"("errin"=w263, "date?"=TRUE, "chaîne"=w265, "in"=w262) -> ("sortie d'erreur"=w260:errorcluster, "refnum en sortie"=w261:refnum<file>)  [unwired: 6 in]
        n110 = local read "BDD"() -> (w254:T2)
        n111 = Bundle By Name(cluster=w254, "Conti"=w246) -> (w253:T2)
        n112 = call "ZenPlusOP600_refaire.vi"("image"="Refaire", "Refaire"=w251, "Cas ok"=OP600ZP_state."CAN Resistance" ("casOK"), "errin"=w247, "test ok ?"=w244) -> ("errout"=w256:errorcluster, "Next"=w250:T7)  [unwired: 5 in]
        n113 = local write "BDD"(w253) -> ()
      }
      frame "CAN Resistance" {
        n114 = call "OUINON.vi"("errin"=w320, "image"="CANRES" ("IN")) -> ("error out"=w319:errorcluster, "OUI/NON"=w318:bool)  [unwired: 8 in]
        n115 = call "Impédance2"("Enable"=w318, "error in (no error)"=w319) -> ("Résistance CAN_BAT / CAN DIAG"=w310:dbl, "Résistance CAN_VEH / CAN SYS"=w313:dbl, "OK"=w315:bool, "error out"=w316:errorcluster)  [unwired: 14 in]
        n116 = Number To Fractional String(number=w313, precision (6)=i16 2 ("précision (6)")) -> (F-format string=w294:string)  [unwired: 2 in]
        n117 = Number To Fractional String(number=w310, precision (6)=i16 2 ("précision (6)")) -> (F-format string=w293:string)  [unwired: 2 in]
        n118 = call "ZenPlusOP600_refaire.vi"("image"="Refaire", "Refaire"=w301, "Cas ok"=OP600ZP_state."VAT" ("casOK"), "errin"=w316, "test ok ?"=w315) -> ("errout"=w298:errorcluster, "Next"=w299:T7)  [unwired: 5 in]
        n119 = local read "BDD"() -> (w296:T2)
        n120 = Bundle By Name(cluster=w296, "VEH_SYS"=w294, "BAT_DIAG"=w293) -> (w295:T2)
        n121 = local write "BDD"(w295) -> ()
        n122 = Concatenate Strings("CAN Resistance;" ("chaîne"), "CAN_VEH / CAN_SYS;" ("chaîne"), w294, ";CAN_BAT / CAN_DIAG;" ("chaîne"), w293) -> (w308:string)
        n123 = call <userlib>:"Log_basic.vi"("errin"=w307, "date?"=TRUE, "chaîne"=w308, "in"=w305) -> ("sortie d'erreur"=w306:errorcluster, "refnum en sortie"=w304:refnum<file>)  [unwired: 6 in]
      }
      frame "Softs" {
        (unwired) TRUE ("Last?")
        # "A réactiver lorsque license sur poste"
        # "C:\\Users\\operateur\\Desktop\\FORSEE Diag tool V1.7.0b8\\FORSEE_Diag.exe"
        # "C:\\Users\\operateur\\Desktop\\synchro_GENII.bat"
        # "Injection des softs (ASW, CONFIG, ASW, APPLI)"
        n124 = disable-structure shown="Désactivé" {
          disable-tunnel: [w342 w344] -> w330
          disable-tunnel: w331 -> [w341 w344]
          frame Disabled {
            # "lancement Synchro_GENII"
            n125 = call "OP600ZP_LaunchEXE.vi"("errin"=w341) -> ("error out"=w343:errorcluster)  [unwired: 8 in]
            n126 = call "OP600ZP_Softs.vi"("errin"=w343) -> ("errout"=w342:errorcluster)  [unwired: 9 in, 1 out]
          }
          frame Enabled {
          }
        }
        n127 = local write "TOP"("Suppression DTC1" ("TOP")) -> ()
        n128 = call "Branche"("error in (no error)"=w330) -> ("n° branche"=w329:dbl, "OK"=w323:bool, "error out"=w326:errorcluster)  [unwired: 16 in]
        n129 = global write "VG_branche.vi" "Branche"(w329) -> ()
        n130 = call "Multi_OUI_NON.vi"("errin"=w326, "errinb"=w323, "Tableau"=string[] ["ALIMON", "MCU_PARK"]) -> ("errout"=w325:errorcluster)  [unwired: 7 in, 1 out]
        n131 = call "DTC_ERASE.vi"("errin"=w325, "UNINIT?"=TRUE) -> ("error out"=w328:errorcluster, "Erased?"=w327:bool)  [unwired: 8 in]
        n132 = call "ZenPlusOP600_refaire.vi"("image"="Refaire", "Refaire"=w334, "Cas ok"=OP600ZP_state."MCU" ("casOK"), "errin"=w328, "test ok ?"=w327) -> ("errout"=w335:errorcluster, "Next"=w332:T7)  [unwired: 5 in]
      }
      frame "MCU" {
        n133 = local write "TOP"("Mesure MCU" ("TOP")) -> ()
        n134 = call <userlib>:"BDD_CHECK_GENERAL.vi"("errin"=w353, "DATA IN"=string[] ["Temperature"] ("Field to select"), "tableName"="TEMP") -> ("errout"=w352:errorcluster, "DATA OUT"=w349:string[][])  [unwired: 7 in]
        n135 = Index Array(array=w349, index (row)=0, index (col)=0 ("disabled index (col)")) -> (element=w346:string)
        n136 = Fract/Exp String To Number(string=w346) -> (number=w345:dbl)  [unwired: 3 in, 1 out]
        n137 = call "OP600ZP_FDT_V2.vi"("errin"=w352, "Tusine"=w345) -> ("errout"=w355:errorcluster, "Log"=w373:string, "is OK?"=w354:bool, "ToBDD"=w366:T13)  [unwired: 6 in]
        n138 = Unbundle(w366) -> (w365:string, w364:string, w363:string, w362:string, w361:string, w360:string, w359:string, w358:string, w357:string, w356:string)
        n139 = local read "BDD"() -> (w368:T2)
        n140 = Bundle By Name(cluster=w368, "PARK_Ubatt"=w365, "PARK_DeltaV"=w364, "PARK_DeltaT"=w363, "PARK_Tmax"=w362, "PARK_Tmin"=w361, "PARK_Vmax"=w360, "PARK_Vmin"=w359, "PARK_Tusine"=w358, "PARK_SOH"=w357, "PARK_SOC"=w356) -> (w367:T2)
        n141 = local write "BDD"(w367) -> ()
        n142 = Concatenate Strings(w373) -> (w372:string)
        n143 = call <userlib>:"Log_basic.vi"("errin"=w381, "date?"=TRUE, "chaîne"=w372, "in"=w380) -> ("sortie d'erreur"=w379:errorcluster, "refnum en sortie"=w378:refnum<file>)  [unwired: 6 in]
        n144 = call "ZenPlusOP600_refaire.vi"("image"="Refaire", "Refaire"=w371, "Cas ok"=OP600ZP_state."Iso" ("Énum"), "errin"=w355, "test ok ?"=w354) -> ("errout"=w374:errorcluster, "Next"=w369:T7)  [unwired: 5 in]
      }
      frame "Iso" {
        # "test d'isolement PDU+, PDU-, bat+et Bat-"
        n145 = call "OUINON.vi"("errin"=w390, "image"="ISOP" ("IN")) -> ("error out"=w398:errorcluster, "OUI/NON"=w397:bool)  [unwired: 8 in]
        n146 = local write "TOP"("Test d'isolement du Pack" ("TOP")) -> ()
        n147 = call "OP600ZP_ISO.vi"("entrée d'erreur (pas d'erreur)"=w398, "Oui"=w397) -> ("sortie d'erreur"=w395:errorcluster, "ISOM"=w383:string, "ISOP"=w384:string, "Booléen"=w393:bool)  [unwired: 6 in]
        n148 = local read "BDD"() -> (w385:T2)
        n149 = Concatenate Strings("Iso+;" ("chaîne"), w384, ";Iso-;" ("chaîne"), w383) -> (w399:string)
        n150 = call "ZenPlusOP600_refaire.vi"("image"="Refaire", "Refaire"=w389, "Cas ok"=OP600ZP_state."OCV" ("casOK"), "errin"=w395, "test ok ?"=w393) -> ("errout"=w394:errorcluster, "Next"=w387:T7)  [unwired: 5 in]
        n151 = Bundle By Name(cluster=w385, "ISOP"=w384, "ISOM"=w383) -> (w386:T2)
        n152 = call <userlib>:"Log_basic.vi"("errin"=w405, "date?"=TRUE, "chaîne"=w399, "in"=w404) -> ("sortie d'erreur"=w406:errorcluster, "refnum en sortie"=w403:refnum<file>)  [unwired: 6 in]
        n153 = local write "BDD"(w386) -> ()
      }
      frame "OCV" {
        # "Attention lors de l'autom, si utilisation du MX5060, risque de dégât matériel si en mauvais position (car utilisé aussi pour Capacité)"
        # "Ratio Ubatt/OCV critère"
        # "OCV critère"
        # "Test OVC et ACIR"
        n154 = call <userlib>:"FGV_Image.vi"("Énum"=FGV."SET", "IN"="OCV") -> ()  [unwired: 9 in, 1 out]
        n155 = call "Mesure OCV"("Enable"=TRUE, "error in (no error)"=w430) -> ("Tension Bat+ Bat- (V)"=w409:dbl, "error out"=w420:errorcluster)  [unwired: 15 in, 1 out]
        n156 = local write "TOP"("Meusure de la tension à vide" ("TOP")) -> ()
        n157 = global read "Ubatt.vi" "Ubatt"() -> (w416:dbl)
        n158 = global write "OCV.vi" "OCV"(w409) -> ()
        n159 = expression code="x+0.02*x"(w416) -> (w423:dbl)
        n160 = expression code="x-0.02*x"(w416) -> (w424:dbl)
        n161 = call <userlib>:"GetP.vi"("errin"=w420, "Pédale ON?"=FALSE) -> ("errout"=w418:errorcluster)  [unwired: 8 in, 1 out]
        n162 = Max & Min(x=w416, y=w409) -> (max(x,y)=w415:dbl, min(x,y)=w414:dbl)
        n163 = In Range and Coerce(upper limit=w423, x=w409, lower limit=w424) -> (In Range?=w422:bool)  [unwired: 1 out]
        n164 = global read "OP600ZP_VGConf.vi" "RatioUBATTOCV"() -> (w417:dbl)
        n165 = Divide(x=w415, y=w414) -> (x/y=w408:dbl)
        n166 = Less Or Equal?(x=w408, y=w417) -> (x <= y?=w413:bool)
        n167 = Compound Arithmetic op=AND ("Opérateur arithmétique")(w422, w413) -> (w421:bool)
        n168 = case shown="True" w421 {
          tunnel: [w439 w452] -> w427
          tunnel: w409 -> [_ w451]
          tunnel: ["0" w450] -> w431
          tunnel: w428 -> [w439 w449]
          tunnel: w426 -> [w440 w448]
          tunnel: [w440 w447] -> w425
          tunnel: w408 -> [_ w442]
          frame False {
          }
          frame True {
            n169 = Number To Decimal String(number=w451, width (-)=i16 2 ("largeur (-)")) -> (decimal integer string=w450:string)
            n170 = Number To Decimal String(number=w442, width (-)=i16 2 ("largeur (-)")) -> (decimal integer string=w445:string)
            n171 = Concatenate Strings("OCV;" ("chaîne"), w450, ";Ratio OCV/Ubatt;" ("chaîne"), w445) -> (w454:string)
            n172 = call <userlib>:"Log_basic.vi"("errin"=w448, "date?"=TRUE, "chaîne"=w454, "in"=w449) -> ("sortie d'erreur"=w447:errorcluster, "refnum en sortie"=w452:refnum<file>)  [unwired: 6 in]
          }
        }
        n173 = local read "BDD"() -> (w433:T2)
        n174 = Bundle By Name(cluster=w433, "OCV"=w431) -> (w432:T2)
        n175 = call "ZenPlusOP600_refaire.vi"("image"="Refaire", "Refaire"=w412, "Cas ok"=OP600ZP_state."DTC" ("Énum"), "errin"=w418, "test ok ?"=w421) -> ("errout"=w429:errorcluster, "Next"=w410:T7)  [unwired: 5 in]
        n176 = local write "BDD"(w432) -> ()
      }
      frame "DTC" {
        (unwired) TRUE ("Last?")
        # "Vérification de l'absence de DTC dans FDT"
        n177 = call "Stall Data Flow.vim"("value in"=w462, "milliseconds to wait"=u32 2000) -> ("value out"=w463:errorcluster)  [unwired: 1 out]
        n178 = call <userlib>:"FGV_Image.vi"("Énum"=FGV."SET", "IN"="DTCERASE") -> ()  [unwired: 9 in, 1 out]
        n179 = local write "TOP"("Vérification absence DTC" ("TOP")) -> ()
        n180 = call "DTC_ERASE.vi"("errin"=w463, "UNINIT?"=TRUE) -> ("error out"=w458:errorcluster, "Erased?"=w457:bool)  [unwired: 8 in]
        n181 = Select(t="NO DTC;", s=w457, f=";DTC DETECTE(S)") -> (s? t:f=w465:string)
        n182 = Concatenate Strings("DTC;" ("chaîne"), w465) -> (w478:string)
        n183 = call <userlib>:"Log_basic.vi"("errin"=w475, "date?"=TRUE, "chaîne"=w478, "in"=w473) -> ("sortie d'erreur"=w474:errorcluster, "refnum en sortie"=w472:refnum<file>)  [unwired: 6 in]
        n184 = call "ZenPlusOP600_refaire.vi"("image"="Refaire", "Refaire"=w470, "Cas ok"=OP600ZP_state."Capacitance" ("casOK"), "errin"=w458, "test ok ?"=w457) -> ("errout"=w479:errorcluster, "Next"=w468:T7)  [unwired: 5 in]
      }
      frame "Capacitance" {
        w489 = 1000.0 ("y")
        w512 = i16 2 ("précision (6)")
        # "Valeur lue MX5060 en uF"
        n185 = call "OUINON.vi"("errin"=w526, "image"="CAPA1" ("IN")) -> ("error out"=w525:errorcluster, "OUI/NON"=w521:bool)  [unwired: 8 in]
        n186 = case shown="True" w521 {
          tunnel: w525 -> [w538 w543]
          tunnel: [w538 w540] -> w523
          tunnel: [FALSE ("Aucun DTC") w541] -> _
          tunnel: [0.0 ("Valeur de la capacité BAT+") w539] -> w490
          frame False {
          }
          frame True {
            n187 = call "Mesure de capacité BAT+"("Enable"=TRUE, "error in (no error)"=w543) -> ("Valeur de la capacité BAT+"=w539:dbl, "OK"=w541:bool, "error out"=w540:errorcluster)  [unwired: 15 in]
          }
        }
        n188 = local write "TOP"("Test de capacité" ("TOP")) -> ()
        n189 = call "OUINON.vi"("errin"=w523, "image"="CAPA2" ("IN")) -> ("error out"=w522:errorcluster, "OUI/NON"=w520:bool)  [unwired: 8 in]
        n190 = case shown="True" w520 {
          tunnel: w522 -> [w530 w535]
          tunnel: [w530 w532] -> w508
          tunnel: [FALSE ("Aucun DTC") w533] -> _
          tunnel: [0.0 ("Valeur de la capacité BAT-") w531] -> w492
          frame False {
          }
          frame True {
            n191 = call "Mesure de capacité BAT-"("Enable"=TRUE, "error in (no error)"=w535) -> ("Valeur de la capacité BAT-"=w531:dbl, "OK"=w533:bool, "error out"=w532:errorcluster)  [unwired: 15 in]
          }
        }
        n192 = global read "OP600ZP_VGConf.vi" "CBAT+"() -> (w495:dbl)
        n193 = global read "OP600ZP_VGConf.vi" "CBAT-"() -> (w498:dbl)
        n194 = Divide(x=w498, y=1000.0) -> (x/y=w497:dbl)
        n195 = Multiply(x=w492, y=w489) -> (x*y=w491:dbl)
        n196 = Multiply(x=w490, y=w489) -> (x*y=w488:dbl)
        n197 = global read "OP600ZP_VGConf.vi" "CBATmin"() -> (w487:dbl)
        n198 = Divide(x=w495, y=1000.0) -> (x/y=w493:dbl)
        n199 = Number To Fractional String(number=w491, precision (6)=w512) -> (F-format string=w481:string)  [unwired: 2 in]
        n200 = Number To Fractional String(number=w488, precision (6)=w512) -> (F-format string=w482:string)  [unwired: 2 in]
        n201 = Divide(x=w487, y=1000.0) -> (x/y=w485:dbl)
        n202 = In Range and Coerce(upper limit=w497, x=w492, lower limit=w485) -> (In Range?=w500:bool)  [unwired: 1 out]
        n203 = In Range and Coerce(upper limit=w493, x=w490, lower limit=w485) -> (In Range?=w499:bool)  [unwired: 1 out]
        n204 = And(x=w500, y=w499) -> (x .and. y?=w507:bool)
        n205 = Concatenate Strings("Capacitance;" ("chaîne"), "CBAT+;" ("chaîne"), w482, ";CBAT-;" ("chaîne"), w481) -> (w514:string)
        n206 = call "ZenPlusOP600_refaire.vi"("image"="Refaire", "Refaire"=w505, "Cas ok"=OP600ZP_state."INTERLOOP" ("casOK"), "errin"=w508, "test ok ?"=w507) -> ("errout"=w506:errorcluster, "Next"=w503:T7)  [unwired: 5 in]
        n207 = call <userlib>:"Log_basic.vi"("errin"=w518, "date?"=TRUE, "chaîne"=w514, "in"=w516) -> ("sortie d'erreur"=w517:errorcluster, "refnum en sortie"=w515:refnum<file>)  [unwired: 6 in]
        n208 = local read "BDD"() -> (w484:T2)
        n209 = Bundle By Name(cluster=w484, "CBAT+"=w482, "CBAT-"=w481) -> (w483:T2)
        n210 = local write "BDD"(w483) -> ()
      }
      frame "INTERLOOP" {
        n211 = local write "TOP"("Test Interlock Loop" ("TOP")) -> ()
        n212 = call "OP600ZP_INTLCK_LOOP.vi"("errin"=w551) -> ("errout"=w550:errorcluster, "pass?"=w544:bool, "Logout"=w546:string)  [unwired: 8 in]
        n213 = case shown="True" w544 {
          tunnel: w550 -> [w566 w569]
          tunnel: [w566 w568] -> w549
          tunnel: [_ w567] -> w545
          frame False {
          }
          frame True {
            n214 = call "OUINON.vi"("errin"=w569, "image"="DTC_DRIVE") -> ("error out"=w572:errorcluster)  [unwired: 8 in, 1 out]
            n215 = flat-sequence {
              tunnel: w572 -> [w578]
              tunnel: [w577] -> w571
              frame #0 {
                n216 = call "Stall Data Flow.vim"("value in"=w578, "milliseconds to wait"=u32 2000) -> ("value out"=w577:errorcluster)  [unwired: 1 out]
                n217 = call <userlib>:"FGV_Image.vi"("Énum"=FGV."SET", "IN"="DTCERASE") -> ()  [unwired: 9 in, 1 out]
              }
            }
            n218 = call "DTC_ERASE.vi"("errin"=w571, "UNINIT?"=TRUE) -> ("error out"=w568:errorcluster, "Erased?"=w567:bool)  [unwired: 8 in]
          }
        }
        n219 = case shown="True" w545 {
          tunnel: ["DTC" "NO DTC"] -> w552
          frame False {
          }
          frame True {
          }
        }
        n220 = case shown="True" w545 {
          tunnel: w549 -> [w579 w583]
          tunnel: [w579 w582] -> w548
          tunnel: [_ w580] -> w547
          frame False {
          }
          frame True {
            n221 = call "OUINON.vi"("errin"=w583, "image"="PARK_PRECHARGE") -> ("error out"=w582:errorcluster, "OUI/NON"=w580:bool)  [unwired: 8 in]
          }
        }
        n222 = Concatenate Strings(w546, w552) -> (w564:string)
        n223 = call <userlib>:"Log_basic.vi"("errin"=w562, "date?"=TRUE, "chaîne"=w564, "in"=w563) -> ("sortie d'erreur"=w561:errorcluster, "refnum en sortie"=w560:refnum<file>)  [unwired: 6 in]
        n224 = call "ZenPlusOP600_refaire.vi"("image"="Refaire", "Refaire"=w557, "Cas ok"=OP600ZP_state."PreCharge" ("casOK"), "errin"=w548, "test ok ?"=w547) -> ("errout"=w555:errorcluster, "Next"=w556:T7)  [unwired: 5 in]
      }
      frame "Current + DCIR" {
        n225 = call "OUINON.vi"("errin"=w648, "image"="DCIR1" ("IN")) -> ("error out"=w646:errorcluster, "OUI/NON"=w647:bool)  [unwired: 8 in]
        n226 = case shown="True" w647 {
          tunnel: w646 -> [w699 w702]
          tunnel: [w699 w701] -> w622
          tunnel: [FALSE ("OUI/NON") w700] -> w593
          frame False {
          }
          frame True {
            n227 = call "OUINON.vi"("errin"=w702, "image"="DCIR2" ("IN")) -> ("error out"=w701:errorcluster, "OUI/NON"=w700:bool)  [unwired: 8 in]
          }
        }
        n228 = global read "PackType.vi" "VG_PackType"() -> (w595:string)
        n229 = local write "TOP"("Test DCIR" ("TOP")) -> ()
        n230 = call "Stall Data Flow.vim"("value in"=w622, "milliseconds to wait"=u32 5000) -> ("value out"=w587:errorcluster)  [unwired: 1 out]
        n231 = case shown="\"ZEN77\", Default" w595 {
          tunnel: [w693 w694 w695 w696 w697] -> w594
          frame "ZEN74" {
            n232 = global read "OP600ZP_VGConf.vi" "Current"() -> (w693:dbl)
          }
          frame "ZEN77", Default {
            n233 = global read "OP600ZP_VGConf.vi" "Current"() -> (w694:dbl)
          }
          frame "ZEN79" {
            n234 = global read "OP600ZP_VGConf.vi" "Current"() -> (w695:dbl)
          }
          frame "ZEN82" {
            n235 = global read "OP600ZP_VGConf.vi" "Current"() -> (w696:dbl)
          }
          frame "ZEN84" {
            n236 = global read "OP600ZP_VGConf.vi" "Current84"() -> (w697:dbl)
          }
        }
        n237 = case shown="True" w593 {
          tunnel: [T1 {"F400 Battery Charge Type"="", "F400 Battery State Request"="", "F400 Ext Insulation Test Control"="", "F400 Int Insulation Test Control"="", "F400 Vehicle Speed"=0, "F400 Ambiant Temperature"=0, "F400 Charger Available Power"=0, "F400 Count"=0, "F106 Keep Active request"="", "F106 Battery State"="", "F106 Operating Status"="", "F106 Battery SOC"=0.0, "F106 Battery SOH"=0.0, "F106 Ext Insulation Test Status"="", "F106 Int Insulation Test Status"="", "F106 Power Distribution Status"="", "F106 Power Switch Off Delay"=0, "F106 Power Switch Off Request"="", "F106 Count"=0, "F101 Battery Voltage"=0, "F101 Battery Current"=0.0, "F101 Max Charge Current"=0, "F101 Max Discharge Current"=0, "F101 Max Discharge Current Temp Limit"="", "F101 Max Discharge Current SOC Limit"="", "F101 Max Charge Current Temp Limit"="", "F101 Max Charge Current SOC Limit"="", "F101 Deliverable Energy"=0.0, "F101 Count"=0, "F102 Cell Average Voltage"=0, "F102 Cell Min Voltage"=0, "F102 Cell Max Voltage"=0, "F103 Cell Average Temp"=0, "F103 Cell Min Temp"=0, "F102 Count"=0, "F103 SumOfInternalResistanceT"=0, "F100 Charge Voltage Setpoint"=0, "F100 Charge Current Setpoint"=0.0, "F100 Equilization Status"=FALSE, "F100 Charge Competed"=FALSE, "F100 Count"=0, "F107 Outlet Water Temp Request"=0, "F107 Outlet Water Temp Status"=0, "F107 Flow Rate Request"=0, "F107 Inlet Water Temp"=0, "F107 Ambiant Temperature 2"=0, "F105 Max Power Charge Continuous"=0, "F105 Max Power Charge Long Prediction"=0, "F105 Max Power Charge Short Prediction"=0, "F105 Max Current Charge Continuous"=0, "F105 Max Current Charge Short Prediction"=0, "F105 Count "=0, "F104 Max Power Discharge Continuous"=0, "F104 Max Power Discharge Long Prediction"=0, "F104 Max Power Discharge Short Prediction"=0, "F104 Max Current Discharge Continuous"=0, "F104 Max Current Discharge Short Prediction"=0, "F104 Count "=0, "F103 Count"=0, "F103 Cell Max Temp"=0, "F103 Max Current Discharge Long Prediction"=0, "F103 Max Current Charge Long Prediction"=0, "F107 Count"=0, "F103 OCV"=0, "F109 DTC"=0} ("cluster de sortie") w715] -> w630
          tunnel: w587 -> [w705 w714]
          tunnel: [w705 w711] -> w609
          tunnel: [FALSE TRUE] -> w608
          frame False {
          }
          frame True {
            # "PREDCIR"
            n238 = call <userlib>:"ZENP_CAN.vi"("Channel No Init"=Channel."PCAN_USBBUS2" ("Channel"), "errin"=w714, "Init?"=TRUE, "uninit?"=TRUE) -> ("errout"=w713:errorcluster, "data out"=w715:T1)  [unwired: 4 in, 1 out]
            n239 = call "Stall Data Flow.vim"("value in"=w713, "milliseconds to wait"=u32 60000) -> ("value out"=w711:errorcluster)  [unwired: 1 out]
          }
        }
        n240 = Unbundle By Name(w630) -> ("F101 Battery Current"=w629:dbl, "F102 Cell Max Voltage"=w628:u32, "F102 Cell Min Voltage"=w627:u32, "F103 Cell Max Temp"=w626:i32, "F103 Cell Min Temp"=w625:i32)
        n241 = case shown="True" w608 {
          tunnel: [w673 w679] -> w589
          tunnel: w609 -> [w673 w678]
          tunnel: w594 -> [_ w689]
          tunnel: ["cluster de sortie 2" w688] -> w592
          tunnel: [w673 w681] -> w590
          tunnel: [FALSE ("30s?") w685] -> w588
          frame False {
          }
          frame True {
            # "23000"
            # "DCIR"
            # "INTRADCIR"
            n242 = global read "VG_ALIM.vi" "ALIM"() -> (w691:string)
            n243 = global read "OP600ZP_VGConf.vi" "Temps"() -> (w675:dbl)
            n244 = property on="progression" class="Slide (strict)"(error in=w678, "Visible"=TRUE) -> ()  [unwired: 1 in, 2 out]
            n245 = call "Stall Data Flow.vim"("value in"=w678, "milliseconds to wait"=u32 23000) -> ("value out"=w686:errorcluster)  [unwired: 1 out]
            n246 = call "OP600_DCIR.vi"("errin"=w678, "Current"=w689, "Durée"=w675, "VISA HITECH"=w691) -> ("errout"=w692:errorcluster, "30s?"=w685:bool)  [unwired: 4 in, 2 out]
            n247 = call <userlib>:"ZENP_CAN.vi"("Channel No Init"=Channel."PCAN_USBBUS2" ("Channel"), "errin"=w686, "Init?"=TRUE, "uninit?"=TRUE) -> ("errout"=w681:errorcluster, "data out"=w688:T1)  [unwired: 4 in, 1 out]
            n248 = call "Stall Data Flow.vim"("value in"=w692, "milliseconds to wait"=u32 500) -> ("value out"=w680:errorcluster)  [unwired: 1 out]
            n249 = call "DCIR_IMAGE.vi"("Time"=w675) -> ()  [unwired: 11 in]
            n250 = property on="progression" class="Slide (strict)"(error in=w680, "Visible"=FALSE) -> (error out=w679:errorcluster)  [unwired: 1 in, 1 out]
          }
        }
        n251 = Subtract(x=w628, y=w627) -> (x-y=w624:u32)
        n252 = Subtract(x=w626, y=w625) -> (x-y=w623:i32)
        n253 = Unbundle By Name(w592) -> ("F101 Battery Voltage"=w617:u32, "F101 Battery Current"=w616:dbl, "F102 Cell Max Voltage"=w621:u32, "F102 Cell Min Voltage"=w620:u32, "F103 Cell Max Temp"=w619:i32, "F103 Cell Min Temp"=w618:i32)
        n254 = Merge Errors(w589, w590) -> (w591:errorcluster)
        n255 = case shown="True" w588 {
          selector: w588 -> [w650 _]
          tunnel: [w651 w656] -> w613
          tunnel: [u32 0 ("F101 Battery Voltage") w668] -> w612
          tunnel: [w650 w667] -> w610
          tunnel: w591 -> [w651 w655]
          frame False {
          }
          frame True {
            # "RELAXATION"
            n256 = property on="progression" class="Slide (strict)"(error in=w655, "Visible"=TRUE) -> (error out=w654:errorcluster)  [unwired: 1 in, 1 out]
            n257 = call "RELAX.vi"() -> ()  [unwired: 12 in]
            n258 = flat-sequence {
              tunnel: [w669] -> w660
              tunnel: w654 -> [w669]
              frame #0 {
                n259 = call <userlib>:"FGV_Image.vi"("Énum"=FGV."SET", "IN"="RELAX") -> ()  [unwired: 9 in, 1 out]
              }
            }
            n260 = call "Stall Data Flow.vim"("value in"=w660, "milliseconds to wait"=u32 30000) -> ("value out"=w659:errorcluster)  [unwired: 1 out]
            n261 = call <userlib>:"ZENP_CAN.vi"("Channel No Init"=Channel."PCAN_USBBUS2" ("Channel"), "errin"=w659, "Init?"=TRUE, "uninit?"=TRUE) -> ("errout"=w666:errorcluster, "data out"=w665:T1)  [unwired: 4 in, 1 out]
            n262 = Unbundle By Name(w665) -> ("F101 Battery Voltage"=w668:u32)
            n263 = call "OP600ZP_Ubatt_Post_Relax.vi"("errin"=w666, "Ubatt Post Relax"=w668) -> ("errout"=w657:errorcluster, "Dans la gamme ?"=w667:bool)  [unwired: 6 in, 2 out]
            n264 = property on="progression" class="Slide (strict)"(error in=w657, "Visible"=FALSE) -> (error out=w656:errorcluster)  [unwired: 1 in, 1 out]
          }
        }
        n265 = Subtract(x=w621, y=w620) -> (x-y=w615:u32)
        "DeltaV30s" <- w615
        n266 = Subtract(x=w619, y=w618) -> (x-y=w614:i32)
        n267 = Bundle("F101 Battery Voltage"=w617, "F101 Battery Current"=w616, w615, w614, "F101 Battery Current"=w629, w624, w623, "F101 Battery Voltage"=w612) -> (w611:T14)  [unwired: 1 in]
        n268 = call "OP600ZP_Assembly.vi"("DCIR_MESURES"=w611) -> ("ToBDD"=w606:T15, "Out"=w634:string, "PASS/FAIL"=w632:bool)  [unwired: 7 in]
        n269 = Unbundle(w606) -> (w604:string, w603:string, w602:string, w601:string, w600:string, w599:string, w598:string, w597:string, w596:string)
        n270 = local read "BDD"() -> (w607:T2)
        n271 = Bundle By Name(cluster=w607, "Post_DCIR_Ubatt"=w604, "Post_DCIR_Current"=w603, "Post_DCIR_DeltaV"=w602, "Post_DCIR_DeltaT"=w601, "Pre_DCIR_Current"=w600, "Pre_DCIR_DeltaV"=w599, "Pre_DCIR_DeltaT"=w598, "Ubatt_PostRelax"=w597, "DCIR@1C"=w596) -> (w605:T2)
        n272 = local write "BDD"(w605) -> ()
        n273 = And(x=w610, y=w632) -> (x .and. y?=w631:bool)
        n274 = call "ZenPlusOP600_refaire.vi"("image"="Refaire", "Refaire"=w643, "Cas ok"=OP600ZP_state."DTC2" ("casOK"), "errin"=w613, "test ok ?"=w631) -> ("errout"=w644:errorcluster, "Next"=w640:T7)  [unwired: 5 in]
        n275 = call <userlib>:"Log_basic.vi"("errin"=w638, "date?"=TRUE, "chaîne"=w634, "in"=w636) -> ("sortie d'erreur"=w637:errorcluster, "refnum en sortie"=w635:refnum<file>)  [unwired: 6 in]
      }
      frame "PreCharge" {
        w749 = 1.0 ("x")
        n276 = call "Multi_OUI_NON.vi"("errin"=w756, "errinb"=TRUE, "Tableau"=string[] ["PRECHARGE1", "PRECHARGE2", "PRE_FUSE"]) -> ("errout"=w732:errorcluster, "isok?"=w733:bool)  [unwired: 7 in]
        n277 = call "PRE_FUSE"("Enable"=w733, "error in (no error)"=w732) -> ("OK"=w734:bool, "error out"=w753:errorcluster)  [unwired: 15 in, 1 out]
        n278 = case shown="True" w734 {
          tunnel: w753 -> [w769 w775]
          tunnel: [w769 w771] -> w752
          tunnel: [FALSE ("OK") w770] -> w727
          frame False {
            (unwired) 0.0 ("Tension")
          }
          frame True {
            n279 = call "OUINON.vi"("errin"=w775, "image"="PRECHARGE3") -> ("error out"=w772:errorcluster, "OUI/NON"=w773:bool)  [unwired: 8 in]
            n280 = call "Tension"("Enable"=w773, "error in (no error)"=w772) -> ("OK"=w770:bool, "error out"=w771:errorcluster)  [unwired: 15 in, 1 out]
          }
        }
        n281 = local write "TOP"("Precharge" ("TOP")) -> ()
        n282 = case shown="True" w727 {
          tunnel: w752 -> [w760 w764]
          tunnel: [w760 w763] -> w721
          tunnel: [0.0 ("Final Voltage :") w762] -> w728
          tunnel: [FALSE ("OK") w761] -> w724
          frame False {
          }
          frame True {
            n283 = call "OUINON.vi"("errin"=w764, "image"="PRECHARGE4") -> ("error out"=w767:errorcluster, "OUI/NON"=w766:bool)  [unwired: 8 in]
            n284 = call "Final Voltage"("Enable"=w766, "error in (no error)"=w767) -> ("Final Voltage :"=w762:dbl, "OK"=w761:bool, "error out"=w763:errorcluster)  [unwired: 15 in]
          }
        }
        n285 = global read "OCV.vi" "OCV"() -> (w750:dbl)
        n286 = Add(x=w749, y=w750) -> (x+y=w751:dbl)
        n287 = Subtract(x=w750, y=w749) -> (x-y=w748:dbl)
        n288 = In Range and Coerce(upper limit=w751, x=w728, lower limit=w748) -> (coerced(x)=w744:dbl, In Range?=w731:bool)
        n289 = And(x=w724, y=w731) -> (x .and. y?=w722:bool)
        n290 = call "Multi_OUI_NON.vi"("errin"=w721, "errinb"=w722, "Tableau"=string[] ["PRECHARGE5", "CAPAOUT"]) -> ("errout"=w719:errorcluster, "isok?"=w720:bool)  [unwired: 7 in]
        n291 = Number To Fractional String(number=w744, precision (6)=i16 2 ("précision (6)")) -> (F-format string=w717:string)  [unwired: 2 in]
        n292 = Concatenate Strings("PreCharge;" ("chaîne"), "VBatterie;" ("chaîne"), ";FinalVoltage;" ("chaîne"), w717) -> (w746:string)
        n293 = call <userlib>:"Log_basic.vi"("errin"=w740, "date?"=TRUE, "chaîne"=w746, "in"=w743) -> ("sortie d'erreur"=w741:errorcluster, "refnum en sortie"=w742:refnum<file>)  [unwired: 6 in]
        n294 = call "ZenPlusOP600_refaire.vi"("image"="Refaire", "Refaire"=w736, "Cas ok"=OP600ZP_state."Current + DCIR" ("casOK"), "errin"=w719, "test ok ?"=w720) -> ("errout"=w737:errorcluster, "Next"=w735:T7)  [unwired: 5 in]
        n295 = local read "BDD"() -> (w718:T2)
        n296 = Bundle By Name(cluster=w718, "FinalVoltage"=w717) -> (w716:T2)
        n297 = local write "BDD"(w716) -> ()
      }
      frame "DTC2" {
        (unwired) TRUE ("Last?")
        n298 = call "DTC_ERASE.vi"("errin"=w780, "UNINIT?"=TRUE) -> ("error out"=w779:errorcluster, "Erased?"=w778:bool)  [unwired: 8 in]
        n299 = Select(t="NO DTC;", s=w778, f=";DTC DETECTE(S)") -> (s? t:f=w777:string)
        n300 = case shown="True" w778 {
          tunnel: [w799 w803] -> w784
          tunnel: [FALSE ("OUI/NON") w802] -> w783
          tunnel: w779 -> [w799 w801]
          frame False {
          }
          frame True {
            n301 = call "OUINON.vi"("errin"=w801, "image"="VAT3" ("IN")) -> ("error out"=w803:errorcluster, "OUI/NON"=w802:bool)  [unwired: 8 in]
          }
        }
        n302 = local write "TOP"("Vérification absence DTC n°2" ("TOP")) -> ()
        n303 = Concatenate Strings("DTC2;" ("chaîne"), w777) -> (w797:string)
        n304 = call <userlib>:"Log_basic.vi"("errin"=w791, "date?"=TRUE, "chaîne"=w797, "in"=w792) -> ("sortie d'erreur"=w788:errorcluster, "refnum en sortie"=w789:refnum<file>)  [unwired: 6 in]
        n305 = call "ZenPlusOP600_refaire.vi"("image"="Refaire", "Refaire"=w793, "Cas ok"=OP600ZP_state."PARK" ("casOK"), "errin"=w784, "test ok ?"=w783) -> ("errout"=w785:errorcluster, "Next"=w787:T7)  [unwired: 5 in]
      }
      frame "PARK" {
        n306 = call "OUINON.vi"("errin"=w824, "image"="POST_FUSE") -> ("error out"=w822:errorcluster, "OUI/NON"=w821:bool)  [unwired: 8 in]
        n307 = call "Poste_Fuse"("Enable"=w821, "error in (no error)"=w822) -> ("OK"=w817:bool, "error out"=w819:errorcluster)  [unwired: 15 in, 1 out]
        n308 = local write "TOP"("Mesure MCU PARK" ("TOP")) -> ()
        n309 = case shown="True" w817 {
          selector: w817 -> [w838 _]
          tunnel: [w838 w847] -> w825
          tunnel: ["" ("Log") w846] -> w820
          tunnel: w819 -> [w840 w845]
          tunnel: [w840 w843] -> w818
          tunnel: [T11 {"", "", "", "", "", "", "", ""} ("ToBDD") w842] -> w815
          frame False {
          }
          frame True {
            n310 = call <userlib>:"ZENP_CAN.vi"("Channel No Init"=Channel."PCAN_USBBUS2" ("Channel"), "errin"=w845) -> ("errout"=w843:errorcluster, "data out"=w844:T1)  [unwired: 6 in, 1 out]
            n311 = call "OP600ZP_FDT_FIN.vi"("Cluster in"=w844) -> ("Log"=w846:string, "is OK?"=w847:bool, "ToBDD"=w842:T11)  [unwired: 8 in]
          }
        }
        n312 = call <userlib>:"Log_basic.vi"("errin"=w830, "date?"=TRUE, "chaîne"=w820, "in"=w829) -> ("sortie d'erreur"=w827:errorcluster, "refnum en sortie"=w826:refnum<file>)  [unwired: 6 in]
        n313 = call "ZenPlusOP600_refaire.vi"("image"="Refaire", "Refaire"=w832, "Cas ok"=OP600ZP_state."FIN_TEST" ("Énum"), "errin"=w818, "test ok ?"=w825) -> ("errout"=w816:errorcluster, "Next"=w831:T7)  [unwired: 5 in]
        n314 = Unbundle(w815) -> (w812:string, w811:string, w810:string, w809:string, w808:string, w807:string, w806:string, w805:string)
        n315 = local read "BDD"() -> (w814:T2)
        n316 = Bundle By Name(cluster=w814, "PARK_DeltaV 2"=w812, "PARK_DeltaT 2"=w811, "PARK_Tmax 2"=w810, "PARK_Tmin 2"=w809, "PARK_Vmax 2"=w808, "PARK_Vmin 2"=w807, "PARK_SOH 2"=w806, "PARK_SOC 2"=w805) -> (w813:T2)
        n317 = local write "BDD"(w813) -> ()
      }
      frame "FIN_TEST" {
        n318 = local write "TOP"("Fin de test" ("TOP")) -> ()
        n319 = call "Multi_OUI_NON.vi"("errin"=w853, "errinb"=TRUE, "Tableau"=string[] ["ETIQ2", "END1", "END2", "END3", "END4", "END5"]) -> ("errout"=w858:errorcluster, "isok?"=w857:bool)  [unwired: 7 in]
        n320 = case shown="True" w857 {
          tunnel: [w864 w875] -> w851
          tunnel: w852 -> [w864 w874]
          tunnel: [w863 w873] -> w848
          tunnel: w850 -> [w863 w872]
          frame False {
          }
          frame True {
            n321 = Concatenate Strings("FIN_TEST;" ("chaîne"), "ETIQ2;" ("chaîne"), "OK;" ("chaîne"), "Esthetique Pack;" ("chaîne"), "OK;" ("chaîne"), "VAT2;" ("chaîne"), "OK" ("chaîne")) -> (w876:string)
            n322 = call <userlib>:"Log_basic.vi"("errin"=w874, "date?"=TRUE, "chaîne"=w876, "in"=w872) -> ("sortie d'erreur"=w875:errorcluster, "refnum en sortie"=w873:refnum<file>)  [unwired: 6 in]
          }
        }
        n323 = call "ZenPlusOP600_refaire.vi"("image"="Refaire", "Refaire"=w855, "Cas ok"=OP600ZP_state."Next" ("casOK"), "errin"=w858, "test ok ?"=w857) -> ("errout"=w849:errorcluster, "Next"=w854:T7)  [unwired: 5 in]
      }
      frame "Crash" {
        # "\\\\forseepower.com\\fr\\040 Production\\FR7 - Poitiers\\06 Production\\05. Electronique\\Documents Control lib\\Archives\\ZEN PLUS"
        n324 = Close File(refnum=w909, error in=w908) -> (path=w879:path, error out=w902:errorcluster)
        n325 = call <userlib>:"FGV_Image.vi"("Énum"=FGV."SET", "IN"="TeamLeader") -> ()  [unwired: 9 in, 1 out]
        n326 = call <userlib>:"waitXms.vi"("attente (ms)"=u32 500, "errin"=w902) -> ("errout"=w895:errorcluster)  [unwired: 13 in]
        n327 = Read from Text File(file (use dialog)=w879, error in=w895) -> (text=w894:string, error out=w892:errorcluster)  [unwired: 2 in, 2 out]
        n328 = call <userlib>:"TEMPS_TEST.vi"("pathin"=w879) -> ("Delay calculé"=w878:string)  [unwired: 9 in, 1 out]
        n329 = case shown="True" TRUE {
          tunnel: [w912 w914] -> w880
          tunnel: w881 -> [w912 w914]
          tunnel: w878 -> [_ w913]
          frame False {
          }
          frame True {
            n330 = local read "BDD"() -> (w917:T2)
            n331 = Bundle By Name(cluster=w917, "Résultat final"="0", "TempsTest"=w913) -> (w915:T2)
            n332 = local write "BDD"(w915) -> ()
          }
        }
        n333 = call "OP600ZP_SN_Reader.vi"("Fichier txt"=w894) -> ("SN"=w887:string)  [unwired: 10 in]
        n334 = local read "BDD"() -> (w889:T2)
        n335 = Unbundle By Name(w889) -> ("PN"=w886:string)
        n336 = Concatenate Strings(w886, "-SN" ("chaîne"), w887) -> (w888:string)
        n337 = call "OP600ZP_NouveauDossier.vi"("entrée d'erreur (pas d'erreur)"=w892, "Nom du repertoire (PN SN)"=w888, "Network before adding a new folder"=path "\\\\forseepower.com\\fr/040 Production/FR7 - Poitiers/06 Production/05. Electronique/Documents Control lib/Archives/ZEN PLUS" ("chemin de la cible (utiliser une boîte de dialogue)")) -> ("sortie d'erreur"=w893:errorcluster, "Network after adding a new folder"=w890:path)  [unwired: 7 in]
        n338 = Copy ("Copier")(8:w893, 10:w890, 11:w879) -> (0:w901:errorcluster)  [unwired: 2 in, 2 out]
        n339 = call "PvgeneratorOP600.vi"("errin"=w901, "network"=w890, "path in"=w879) -> ("sortie d'erreur"=w905:errorcluster, "network out"=w904:path)  [unwired: 5 in, 2 out]
        n340 = Select ("Sélectionner")(t="1", s=FALSE ("sélecteur"), f="0" ("cas faux")) -> (s? t:f=w897:string)
        n341 = call <userlib>:"POP_GOOGLE.vi"("error in"=w905, "chemin"=w904) -> ("error out"=w884:errorcluster)  [unwired: 8 in, 1 out]
        n342 = local read "BDD"() -> (w900:T2)
        n343 = Bundle By Name(cluster=w900, "Résultat final"=w897) -> ()  [unwired: 1 out]
        n344 = flat-sequence {
          tunnel: [TRUE] -> w910
          tunnel: w884 -> [_]
          frame #0 {
          }
        }
      }
      frame "Next" {
        w943 = OP600ZP_state."Null"  # Énum
        w944 = OP600ZP_state."Scan"  # Énum
        # "\\\\forseepower.com\\fr\\040 Production\\FR7 - Poitiers\\06 Production\\05. Electronique\\Documents Control lib\\Archives\\ZEN PLUS"
        n345 = Close File(refnum=w946, error in=w945) -> (path=w920:path, error out=w919:errorcluster)
        n346 = call <userlib>:"waitXms.vi"("attente (ms)"=u32 500, "errin"=w919) -> ("errout"=w939:errorcluster)  [unwired: 13 in]
        n347 = Read from Text File(file (use dialog)=w920, error in=w939) -> (text=w937:string, error out=w936:errorcluster)  [unwired: 2 in, 2 out]
        n348 = call <userlib>:"TEMPS_TEST.vi"("errin"=w919, "pathin"=w920) -> ("Delay calculé"=w918:string)  [unwired: 8 in, 1 out]
        n349 = case shown="True" TRUE {
          tunnel: [w949 w954] -> w924
          tunnel: w923 -> [w949 w954]
          tunnel: w918 -> [_ w950]
          frame False {
          }
          frame True {
            n350 = local read "BDD"() -> (w953:T2)
            n351 = Bundle By Name(cluster=w953, "Résultat final"="1", "TempsTest"=w950) -> (w951:T2)
            n352 = local write "BDD"(w951) -> ()
          }
        }
        n353 = local read "BDD"() -> (w932:T2)
        n354 = call "OP600ZP_SN_Reader.vi"("Fichier txt"=w937) -> ("SN"=w929:string)  [unwired: 10 in]
        n355 = Unbundle By Name(w932) -> ("PN"=w931:string)
        n356 = Concatenate Strings(w931, "-SN" ("chaîne"), w929) -> (w928:string)
        n357 = call "OP600ZP_NouveauDossier.vi"("entrée d'erreur (pas d'erreur)"=w936, "Nom du repertoire (PN SN)"=w928, "Network before adding a new folder"=path "\\\\forseepower.com\\fr/040 Production/FR7 - Poitiers/06 Production/05. Electronique/Documents Control lib/Archives/ZEN PLUS" ("chemin de la cible (utiliser une boîte de dialogue)")) -> ("sortie d'erreur"=w935:errorcluster, "Network after adding a new folder"=w933:path)  [unwired: 7 in]
        n358 = call "OUINON.vi"("errin"=w924, "image"="Next" ("IN")) -> ("error out"=w927:errorcluster, "OUI/NON"=w947:bool)  [unwired: 8 in]
        n359 = local read "BDD"() -> (w921:T2)
        n360 = Copy ("Copier")(8:w935, 10:w933, 11:w920) -> (0:w938:errorcluster)  [unwired: 2 in, 2 out]
        n361 = call "PvgeneratorOP600.vi"("errin"=w938, "BDD"=w921, "network"=w933, "path in"=w920) -> ("sortie d'erreur"=w941:errorcluster, "network out"=w940:path)  [unwired: 4 in, 2 out]
        n362 = call <userlib>:"POP_GOOGLE.vi"("error in"=w941, "chemin"=w940) -> ("error out"=w926:errorcluster)  [unwired: 8 in, 1 out]
        n363 = Select(t=w944, s=w947, f=w943) -> (s? t:f=w925:T7)
      }
      frame "Comext" {
        n364 = disable-structure shown="Disabled" {
          disable-tunnel: w965 -> [w979 _]
          disable-tunnel: w964 -> [w978 _]
          disable-tunnel: [w977 _] -> w963
          disable-tunnel: w962 -> [w976 _]
          disable-tunnel: [w975 _] -> w961
          disable-tunnel: w960 -> [w974 _]
          disable-tunnel: w959 -> [w972 _]
          disable-tunnel: [w970 _] -> w958
          disable-tunnel: w957 -> [w969 _]
          disable-tunnel: [w967 _] -> w956
          disable-tunnel: [w966 _] -> w955
          frame Disabled {
            n365 = call "OUINON.vi"("errin"=w972, "image"="Comext" ("IN")) -> ("error out"=w971:errorcluster, "OUI/NON"=w968:bool)  [unwired: 8 in]
            n366 = case shown="True" w968 {
              tunnel: w979 -> [w984 w997]
              tunnel: w978 -> [w983 w996]
              tunnel: [w983 w995] -> w967
              tunnel: [w984 w994] -> w977
              tunnel: [OP600ZP_state."Crash" ("OUT") w993] -> w966
              tunnel: w976 -> [_ w992]
              tunnel: [w981 w991] -> w975
              tunnel: w974 -> [_ w990]
              tunnel: w971 -> [w981 w989]
              tunnel: [w982 w988] -> w970
              tunnel: w969 -> [w982 w988]
              frame False {
              }
              frame True {
                w985 = OP600ZP_state."Scan"  # Énum
                (unwired) "Comext;" ("testname")
                n367 = local read "PN"() -> (w1008:string)
                n368 = call <vilib>:"Application Directory.vi"() -> ("Application Directory"=w1010:path)
                n369 = call <userlib>:"Read_Param.vi"("Énum"=enum16{"STR", "DBL", "U32"}."U32", "errin"=w989, 9:w1010, "section"="DataDyn", "key"=w1008) -> ("error out"=w1003:errorcluster, "U32"=w1006:u32)  [unwired: 2 in, 3 out]
                n370 = call <userlib>:"FGV_Image.vi"("Énum"=FGV."SET", "IN"="DataDyn") -> ()  [unwired: 9 in, 1 out]
                n371 = property on="progression" class="Slide (strict)"(error in=w1003, "Visible"=TRUE, "Value"=u8 0 ("progression")) -> (error out=w1002:errorcluster)  [unwired: 1 in, 1 out]
                n372 = call "SCAN CMU.vi"("errin"=w1002, "Nb modules"=w1006) -> ("errout"=w1020:errorcluster, "# température + #tension OK?"=w1015:bool, "Vmin"=w1019:dbl, "Vmax"=w1018:dbl, "Tmin"=w1016:dbl, "Tmax"=w1017:dbl)  [unwired: 4 out]
                n373 = call "OP500ZP_Test_DataDyn.vi"("Vcell Max (V)"=w1018, "MCU"=w1015, "Vcell Min (V)"=w1019, "appdir"=w990, "errin"=w1020, "Température usine (°C)"=21.0, "Tcell Max (°C)"=w1017, "Tcell Min (°C)"=w1016) -> ("errout"=w1014:errorcluster, "datalog"=w1022:string, "pass"=w1013:bool)  [unwired: 1 out]
                n374 = call <userlib>:"Log_basic.vi"("errin"=w997, "date?"=TRUE, "chaîne"=w1022, "in"=w996) -> ("sortie d'erreur"=w994:errorcluster, "refnum en sortie"=w995:refnum<file>)  [unwired: 6 in]
                n375 = call "ZenPlusOP600_refaire.vi"("image"="Refaire", "Refaire"=w992, "Pédale"=FALSE, "Cas ok"=w985, "errin"=w1014, "test ok ?"=w1013) -> ("errout"=w998:errorcluster, "Next"=w993:T7)  [unwired: 4 in]
                n376 = property on="progression" class="Slide (strict)"(error in=w998, "Visible"=FALSE, "Value"=u8 0 ("progression")) -> (error out=w991:errorcluster)  [unwired: 1 in, 1 out]
              }
            }
          }
          frame Enabled {
          }
        }
      }
    }
    n377 = Wait (ms)(milliseconds to wait=u32 200 ("attente (ms)")) -> ()  [unwired: 1 out]
    n378 = case shown="True" w62 {
      selector: w62 -> [_ w1023]
      frame False {
      }
      frame True {
        n379 = local write "STOP"(w1023) -> ()
      }
    }
  }
  n380 = Stop(stop? (T)=w12) -> ()
  n381 = call <userlib>:"PEAK_Init_plus.vi"("errin"="errin", "Channel"=Channel."PCAN_USBBUS1", "BTR0BTR1"=BaudrateEenum."CAN_BAUD_500K") -> ("errout"=w5:errorcluster, "Channel out"=w1:T4)  [unwired: 7 in]
  n382 = while {
    shift-right: [w1034] -> w7
    shift-left: "errin" -> [w1035]
    tunnel: w1 -> [w1030]
    i -> [w1032]
    stop <- w1029 stop-if-true
    # "COMMANDE"
    n383 = global read "VG_branche.vi" "Branche"() -> (w1031:dbl)
    n384 = case shown="5" w1031 {
      tunnel: [1025 1026 1027 1028 1029 u32 1024 ("Identifier")] -> w1037
      frame 2 {
      }
      frame 3 {
      }
      frame 4 {
      }
      frame 5 {
      }
      frame 6 {
      }
      frame 1, Default {
      }
    }
    n385 = case shown="2" "O/P/D" {
      tunnel: [1 2 0] -> w1027
      frame 1 {
      }
      frame 2 {
      }
      frame 0, Default {
      }
    }
    n386 = call "Stall Data Flow.vim"("value in"=w1035, "milliseconds to wait"=u32 100) -> ("value out"=w1033:errorcluster)  [unwired: 1 out]
    n387 = Quotient & Remainder(x=w1032, y=15) -> (x-y*floor(x/y)=w1040:i32)  [unwired: 1 out]
    n388 = Replace Array Subset(array=i32[] [0, 0, 0, 65, 254, 0, 0, 0], new element #1=w1040, index #1=5 ("indice"), new element #2=w1027, index #2=0 ("indice")) -> (w1028:i32[])
    n389 = call <userlib>:"PEAK_Can_Write.vi"("CAN handle"=w1030, "errin"=w1033, "CAN Data"=w1028, "Identifier"=w1037) -> ("errout"=w1034:errorcluster)  [unwired: 7 in]
    n390 = global read "VG_Stop" "Stop?"() -> (w1029:bool)
    n391 = case shown="1" w1027 {
      tunnel: [w1044 w1046 TRUE] -> w1024
      tunnel: [TRUE w1046 w1048] -> w1025
      tunnel: [w1044 TRUE w1048] -> w1026
      frame 1 {
        w1044 = FALSE
      }
      frame 2 {
        w1046 = FALSE
      }
      frame 0, Default {
        w1048 = FALSE
      }
    }
    "OFF" <- w1024
    "PARK" <- w1025
    "DRIVE" <- w1026
  }
  n392 = while {
    tunnel: w5 -> [w1075]
    tunnel: w1 -> [w1074]
    tunnel: [w1059] -> w8
    stop <- w1064 stop-if-true
    # "TROUVER COMMENT EXPLOITER"
    n393 = call <userlib>:"PEAK_Can_Write.vi"("CAN handle"=w1074, "MSG type"=enum8{"STD", "RTR", "XTD", "XTD RTR", "STATUS"}."XTD", "errin"=w1075, "CAN Data"=u8[] [1, 0, 0, 0, 0, 0, 0, 0], "Identifier"=u32 419401608) -> ("errout"=w1063:errorcluster)  [unwired: 6 in]
    n394 = global read "VG_branche.vi" "Branche"() -> (w1067:dbl)
    n395 = call "Stall Data Flow.vim"("value in"=w1063, "milliseconds to wait"=u32 100) -> ("value out"=w1062:errorcluster)  [unwired: 1 out]
    n396 = call <userlib>:"PEAK_Can_Read.vi"("errin"=w1062, "Channel out"=w1074) -> ("errout"=w1059:errorcluster, "MessageBuffer out"=w1069:T16)  [unwired: 7 in, 1 out]
    n397 = Unbundle By Name(w1069) -> ("ID"=w1070:u32)
    n398 = case shown="2" w1067 {
      tunnel: w1070 -> [w1082 w1087 w1093 w1098 w1102 w1109]
      tunnel: w1069 -> [w1084 w1089 w1094 w1099 w1104 w1108]
      tunnel: [w1083 w1088 w1092 w1097 w1103 w1107] -> w1065
      frame 2 {
        n399 = case shown="116" w1082 {
          tunnel: [T16 {"ID"=0, "MSGTYPE"=0, "LEN"=0, "DATA[0]"=0, "DATA[1]"=0, "DATA[2]"=0, "DATA[3]"=0, "DATA[4]"=0, "DATA[5]"=0, "DATA[6]"=0, "DATA[7]"=0} ("MessageBuffer out") w1086] -> w1083
          tunnel: w1084 -> [_ w1086]
          frame 0, Default {
          }
          frame 278 {
          }
        }
      }
      frame 3 {
        n400 = case shown="0, Default" w1087 {
          tunnel: [T16 {"ID"=0, "MSGTYPE"=0, "LEN"=0, "DATA[0]"=0, "DATA[1]"=0, "DATA[2]"=0, "DATA[3]"=0, "DATA[4]"=0, "DATA[5]"=0, "DATA[6]"=0, "DATA[7]"=0} ("MessageBuffer out") w1091] -> w1088
          tunnel: w1089 -> [_ w1091]
          frame 0, Default {
          }
          frame 294 {
          }
        }
      }
      frame 4 {
        n401 = case shown="0, Default" w1093 {
          tunnel: [T16 {"ID"=0, "MSGTYPE"=0, "LEN"=0, "DATA[0]"=0, "DATA[1]"=0, "DATA[2]"=0, "DATA[3]"=0, "DATA[4]"=0, "DATA[5]"=0, "DATA[6]"=0, "DATA[7]"=0} ("MessageBuffer out") w1096] -> w1092
          tunnel: w1094 -> [_ w1096]
          frame 0, Default {
          }
          frame 310 {
          }
        }
      }
      frame 5 {
        n402 = case shown="146" w1098 {
          tunnel: [T16 {"ID"=0, "MSGTYPE"=0, "LEN"=0, "DATA[0]"=0, "DATA[1]"=0, "DATA[2]"=0, "DATA[3]"=0, "DATA[4]"=0, "DATA[5]"=0, "DATA[6]"=0, "DATA[7]"=0} ("MessageBuffer out") w1101] -> w1097
          tunnel: w1099 -> [_ w1101]
          frame 0, Default {
          }
          frame 326 {
          }
        }
      }
      frame 6 {
        n403 = case shown="0, Default" w1102 {
          tunnel: [T16 {"ID"=0, "MSGTYPE"=0, "LEN"=0, "DATA[0]"=0, "DATA[1]"=0, "DATA[2]"=0, "DATA[3]"=0, "DATA[4]"=0, "DATA[5]"=0, "DATA[6]"=0, "DATA[7]"=0} ("MessageBuffer out") w1106] -> w1103
          tunnel: w1104 -> [_ w1106]
          frame 0, Default {
          }
          frame 262 {
          }
        }
      }
      frame 1, Default {
        n404 = case shown="0, Default" w1109 {
          tunnel: [T16 {"ID"=0, "MSGTYPE"=0, "LEN"=0, "DATA[0]"=0, "DATA[1]"=0, "DATA[2]"=0, "DATA[3]"=0, "DATA[4]"=0, "DATA[5]"=0, "DATA[6]"=0, "DATA[7]"=0} ("MessageBuffer out") w1111] -> w1107
          tunnel: w1108 -> [_ w1111]
          frame 0, Default {
          }
          frame 262 {
          }
        }
      }
    }
    n405 = global read "VG_Stop" "Stop?"() -> (w1064:bool)
    n406 = call <userlib>:"DATA_SELECT.vi"("106"=w1065) -> ("106"=w1066:u8[])  [unwired: 10 in, 4 out]
    n407 = call "CAN_READ_SK.vi"("ID106"=w1066) -> ("cluster de sortie"=w1068:T1)  [unwired: 14 in]
    n408 = Unbundle By Name(w1068) -> ("F106 Battery State"=w1060:string)
    n409 = case shown="\"O\", Default" w1060 {
      tunnel: [w1076 w1078 TRUE] -> _
      tunnel: [TRUE w1078 w1080] -> _
      tunnel: [w1076 TRUE w1080] -> _
      frame "1" {
        w1076 = FALSE
      }
      frame "2" {
        w1078 = FALSE
      }
      frame "O", Default {
        w1080 = FALSE
      }
    }
  }
  "error out" <- w8
  n410 = Merge Errors(w28, w27) -> (→"errout":errorcluster)
  n411 = call <userlib>:"CAN Uninitialize.vi"("error in (no error)"=w7, "Channel"=Channel."PCAN_USBBUS1") -> ()  [unwired: 7 in, 3 out]
  n412 = disable-structure shown="Activé" {
    disable-tunnel: [w1112 _] -> _
    frame Disabled {
      n413 = call "Data Dynamiques"() -> ("CMU OK"=w1112:bool)  [unwired: 12 in, 7 out]
    }
    frame Enabled {
    }
  }
  "STOP" <- w25
